vi "Pressures_Low_Server.vi"(0 "Serial port":refnum<visa-resource-name>="COM1", 1 "Commands":T2[](array[typedef]), 5 "Data rate (Hz)":dbl=100.0, 7 "Max. num. sensors (override)":u8=64 max=64, 9 "Wait for HW trigger":bool, 11 "Finite samples":bool=TRUE, 12 "N samples":u32=1000, 14 "Error in":errorcluster) -> (4 "P data (mode 0)":T8[](array[typedef]), 15 "Error out":errorcluster)   [LabVIEW 2020]
doc: "User interface for 64 pressure multiplexer system designed by Paul Nathan, 02/2016"
uses:
  Ctls/System status.ctl
  Ctls/Environmental state values.ctl
  Ctls/Inertial state values.ctl
  Ctls/AccelGyro constants.ctl
  Ctls/Pressure sensor constants.ctl
  Ctls/Cmd list.ctl
  Ctls/Data values, Mode 0 (for datalog).ctl
  Ctls/All state values (for datalog).ctl
  Ctls/Cmd str.ctl
  Ctls/Data values, Mode 1 (for datalog).ctl
  Pressure_Multiplexer_Server_Global.vi
panel:
  in  "Main tabs":T1(tab)
  in  "Env. period (ms)":i32=1000 min=0
  out "Command":T2
  out "ACK 8":bool caption="ACK"
  out "ACK 7":bool caption="ACK"
  out "ACK 6":bool caption="ACK"
  out "AccelGyro constants":T3={"gyrRange"=125.0, "accRange"=2.0, "gx offset"=0.0, "gy offset"=0.0, "gz offset"=0.0, "ax offset"=0.0, "ay offset"=0.0, "az offset"=0.0, "axyz scale"=1.0} {"axyz scale" format="%#_4f"; "az offset" format="%#_4f"; "ay offset" format="%#_4f"; "ax offset" format="%#_4f"; "gz offset" format="%#_4f"; "gy offset" format="%#_4f"; "gx offset" format="%#_4f"; "gyrRange" format="%#_4f"; "accRange" format="%#_4f"}
  out "Faulty sensors":i32[](array[numeric])
  out "ACK 5":bool caption="ACK"
  out "Active sensors":i32[](array[numeric])
  out "ACK 4":bool caption="ACK"
  in  "Gyro. rate (Hz)":u8(ring) items=["6.25", "12.5", "25", "50", "100", "200", "400", "800", "1600", "3200"]
  in  "Gyro. range (dps)":u8(ring) items=["+/- 125", "+/- 250", "+/- 500", "+/- 1000", "+/- 2000"]
  in  "Accel. rate (Hz)":u8(ring)=1 items=["3.125", "6.25", "12.5", "25", "50", "100", "200", "400", "800", "1600"]
  in  "Accel. range (g)":u8(ring) items=["+/- 2", "+/- 4", "+/- 8", "+/- 16"]
  out "Inertial state values":T4 {"w_z (dps)" format="%#_4f"; "a_y (g)" format="%#_4f"; "a_z (g)" format="%#_4f"; "w_y (dps)" format="%#_4f"; "a_x (g)" format="%#_4f"; "Sensor temp. (degC)" format="%#.2f"; "w_x (dps)" format="%#_4f"}
  out "Environmental state values":T5 {"Dew point (degC)" format="%#.2f"; "Density (kg/m^3)" format="%#.3f"; "Pressure alt. (m)" format="%#.2f"; "Density alt. (m)" format="%#.2f"; "Rel. Humidity (%)" format="%#.2f"; "P_atmos (Pa)" format="%#_6f"; "Sensor temp. (degC)" format="%#.2f"; "Thermistor (degC)" format="%#.2f"}
  out "System status":T6
  out "ACK 3":bool caption="ACK"
  out "ACK 1":bool caption="ACK"
  in  "Data mode":u8(ring) items=["P", "P & T"]
  out "ACK 2":bool caption="ACK"
  out "Main Power":bool
  out "L_data (bytes)":u16
  out "Serial no.":u16 format="%04x"
  out "Active pressure sensor constants":T7[](array[typedef])
  out "No Of Channels":i32=1000
  out "Streaming":bool
  out "Clock drift":bool
  out "Sensor temperatures time trace (Mode \"P & T\" only)":sgl[][](graph)
  out "Pressures time trace":sgl[][](graph)
  in  "Stop streaming":bool
  out "Stale samples flag":u8[][](graph)
  out "Samples acquired":u32
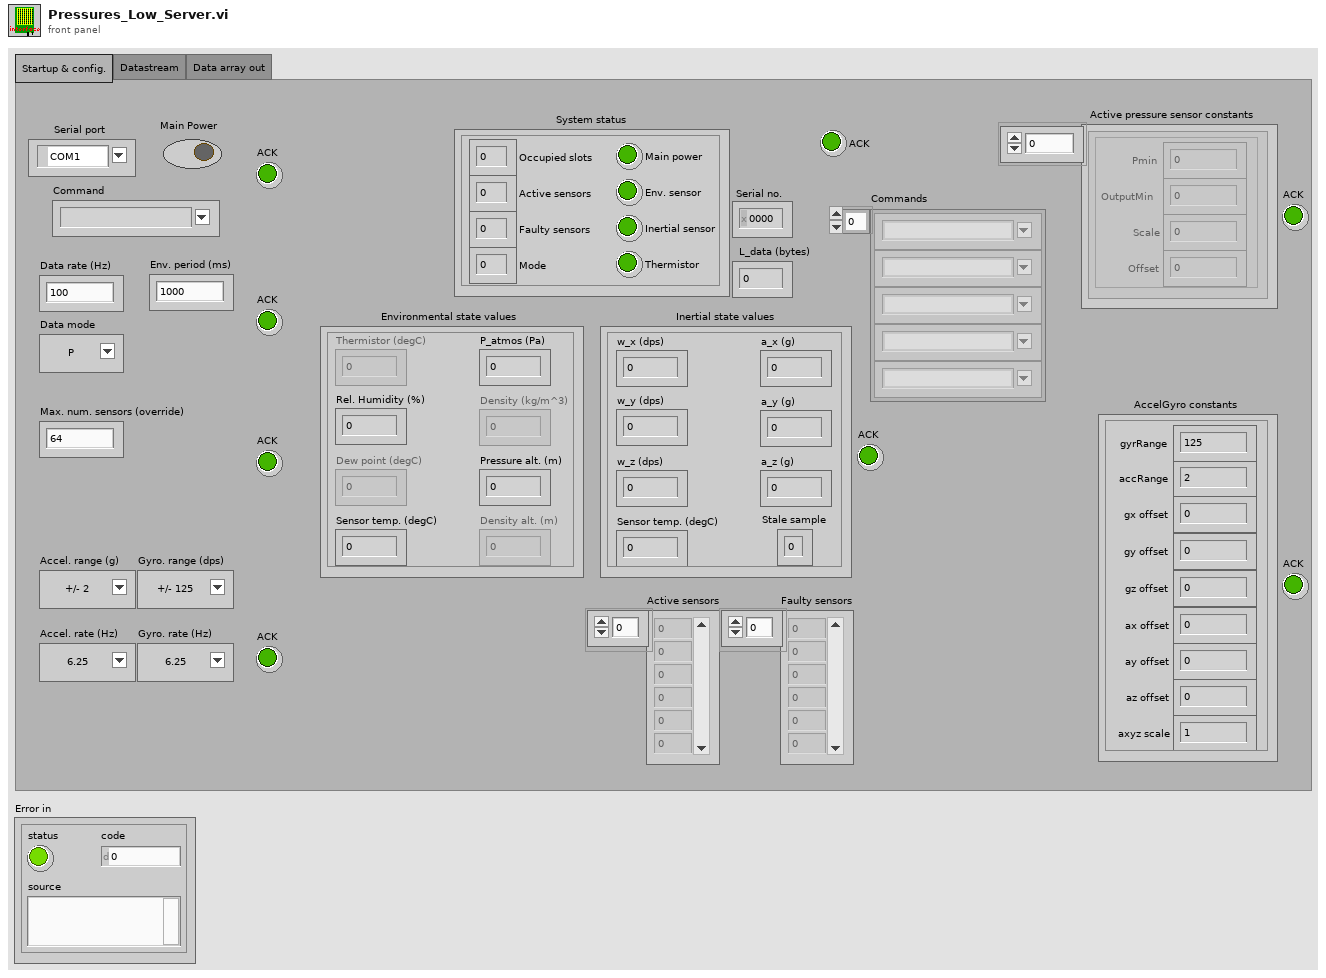
[diagram p1: front panel]
types:
  T1 = enum32{"Startup & config.", "Datastream", "Data array out"}
  T2 = typedef "Cmd list.ctl" = string
  T3 = typedef "AccelGyro constants.ctl" = cluster{"gyrRange":sgl, "accRange":sgl, "gx offset":sgl, "gy offset":sgl, "gz offset":sgl, "ax offset":sgl, "ay offset":sgl, "az offset":sgl, "axyz scale":sgl}
  T4 = typedef "Inertial state values.ctl" = cluster{"w_x (dps)":sgl, "w_y (dps)":sgl, "w_z (dps)":sgl, "a_x (g)":sgl, "a_y (g)":sgl, "a_z (g)":sgl, "Stale sample":u8, "Sensor temp. (degC)":sgl}
  T5 = typedef "Environmental state values.ctl" = cluster{"Thermistor (degC)":sgl, "Sensor temp. (degC)":sgl, "P_atmos (Pa)":sgl, "Rel. Humidity (%)":sgl, "Density (kg/m^3)":sgl, "Dew point (degC)":sgl, "Pressure alt. (m)":sgl, "Density alt. (m)":sgl}
  T6 = typedef "System status.ctl" = cluster{"Main power":bool, "Occupied slots":u8, "Active sensors":u8, "Faulty sensors":u8, "Env. sensor":bool, "Inertial sensor":bool, "Thermistor":bool, "Mode":u8}
  T7 = typedef "Pressure sensor constants.ctl" = cluster{"Pmin":sgl, "OutputMin":sgl, "Scale":sgl, "Offset":sgl}
  T8 = typedef "Data values, Mode 0 (for datalog).ctl" = cluster{"Time Stamp":timestamp, "dt (us)":sgl, "dt_warn":u8, "Pressures":sgl[], "Statuses":u8[]}
  T9 = typedef "All state values (for datalog).ctl" = cluster{"Time Stamp":timestamp, "dt (ms)":i32, "Environmental state values":T5, "Inertial state values":T4}
  T10 = typedef "Cmd str.ctl" = string
  T11 = typedef "Data values, Mode 1 (for datalog).ctl" = cluster{"Time Stamp":timestamp, "dt (us)":sgl, "dt_warn":u8, "Pressures":sgl[], "Die temps.":sgl[], "Statuses":u8[]}
  T12 = enum8{"Enabled", "Disabled", "Disabled and Grayed Out"}
  T13 = typedef "Rendezvous RefNum" = refnum<k1>
  T14 = typedef "EEPROM page.ctl" = cluster{"Pmin (Pa)":sgl, "Pmax (Pa)":sgl, "maxCount":u16, "minCount":u16, "Poffset (Pa)":sgl}
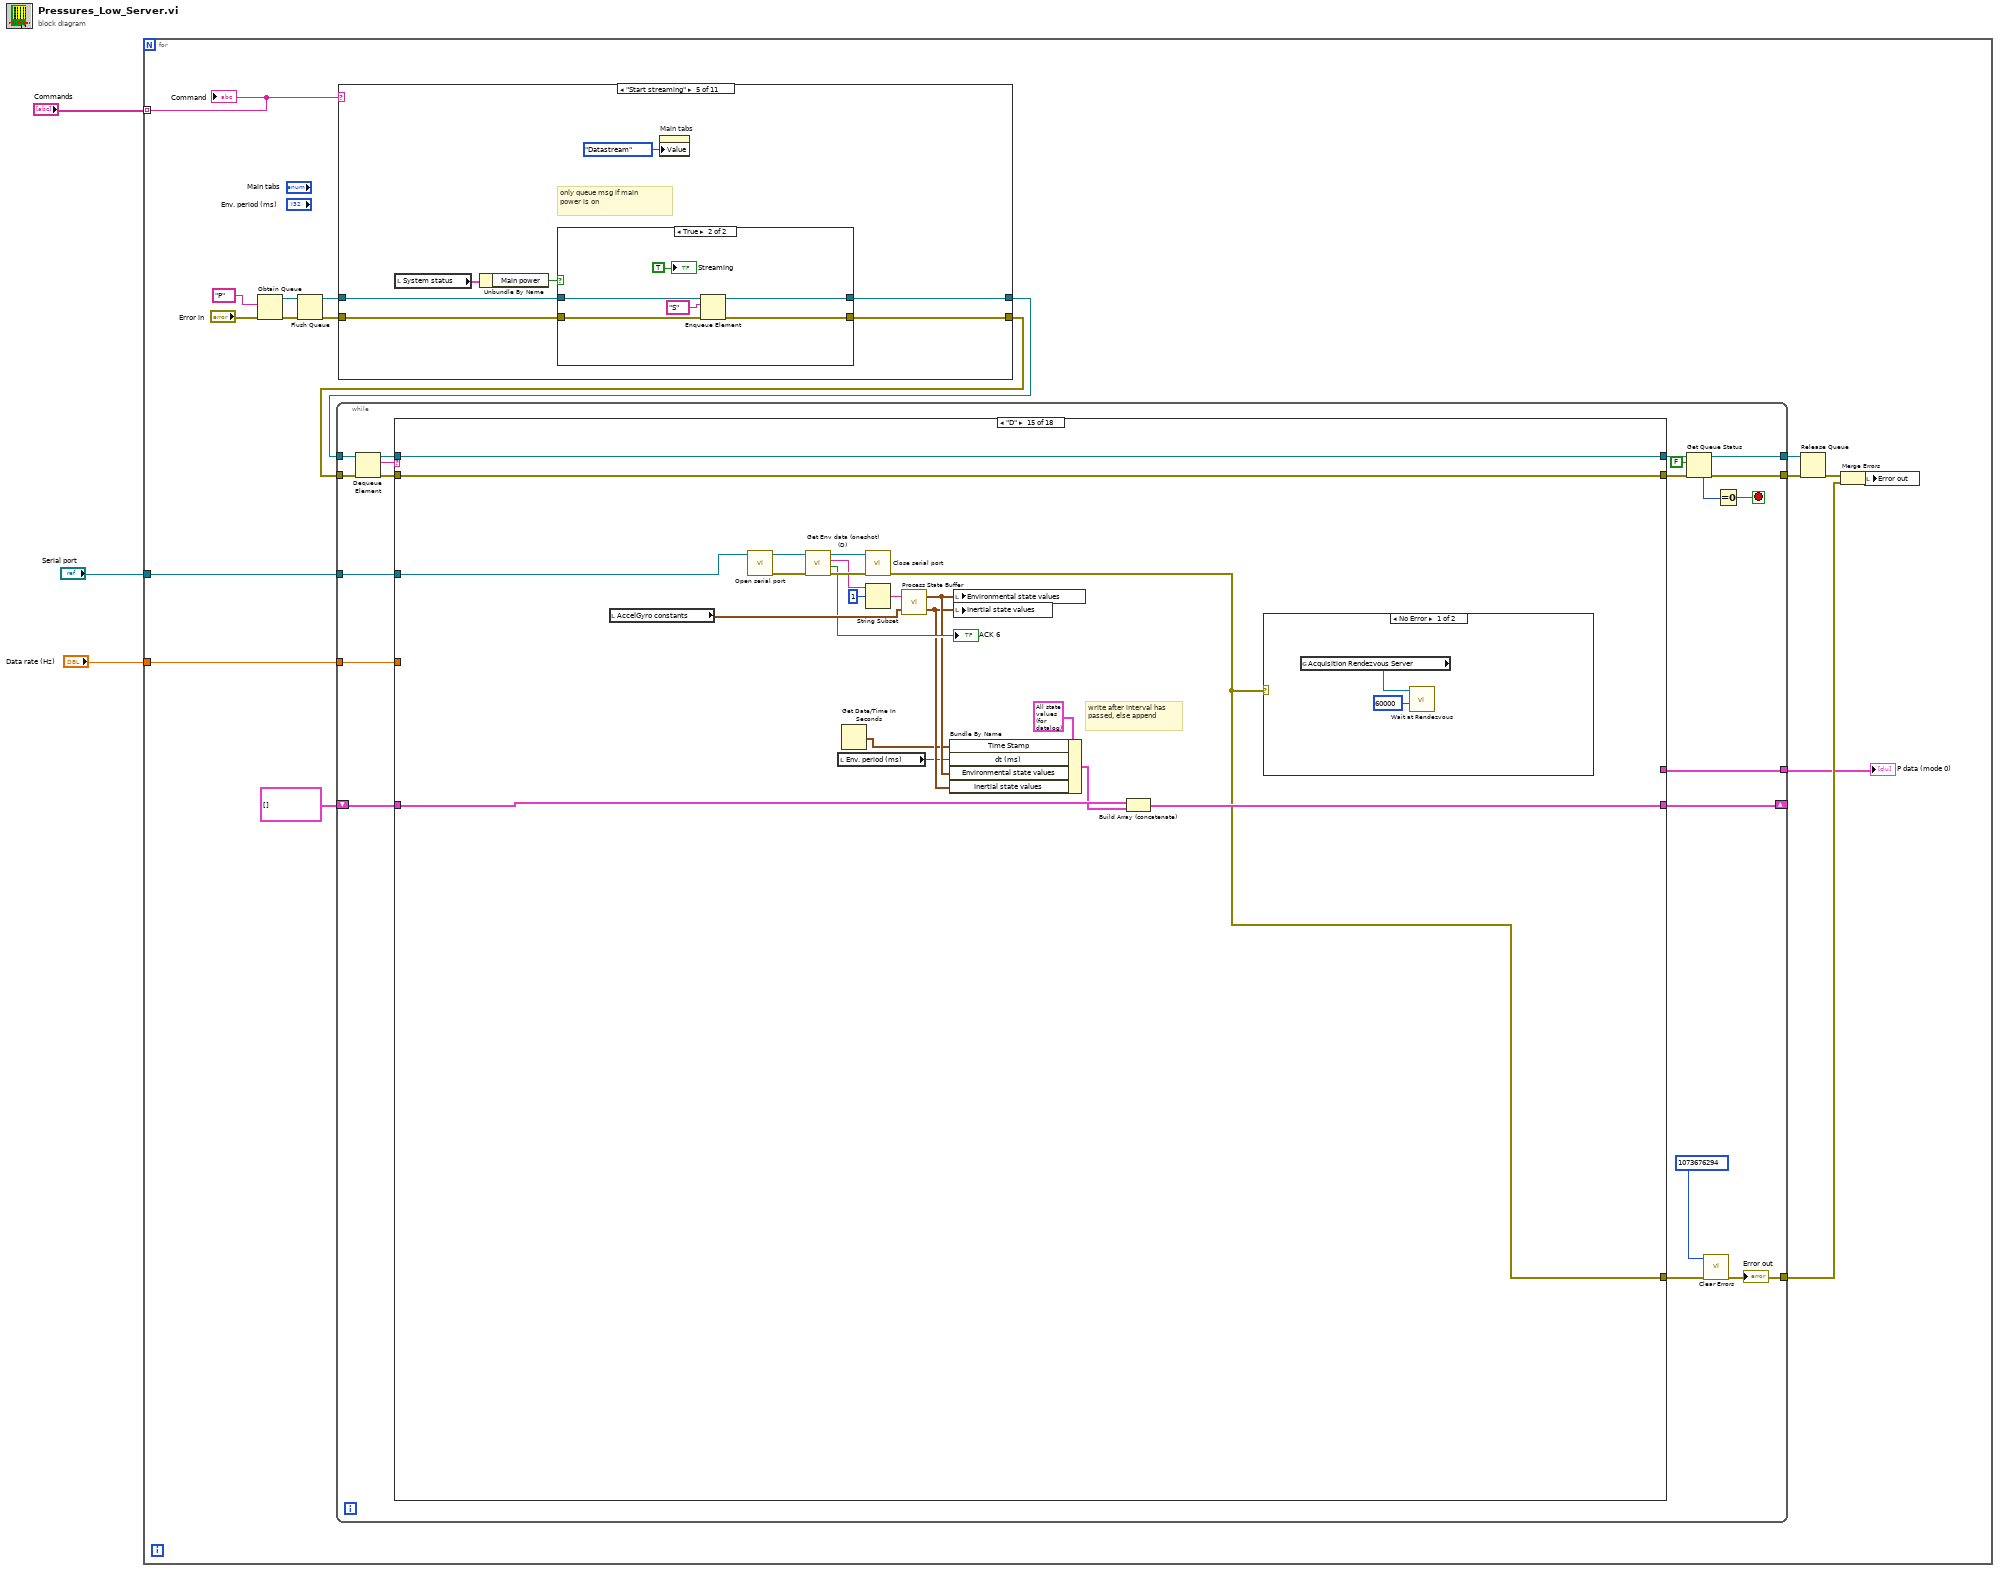
[diagram p0: block diagram]
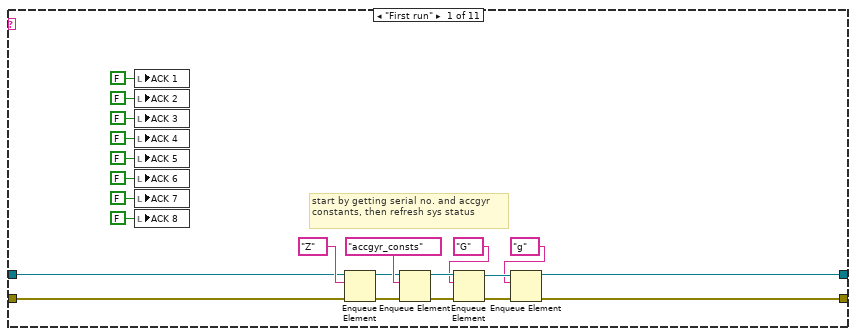
[diagram p2: hidden frame]
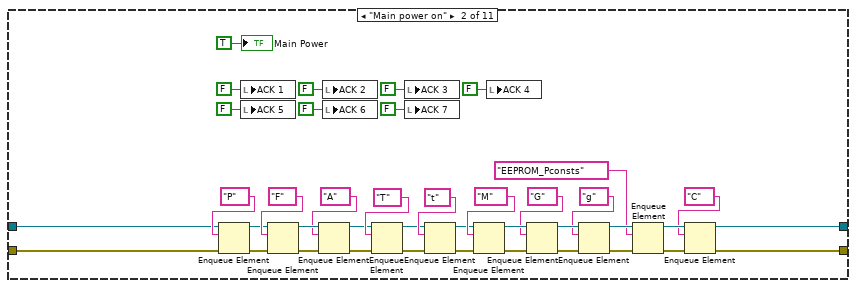
[diagram p3: hidden frame]
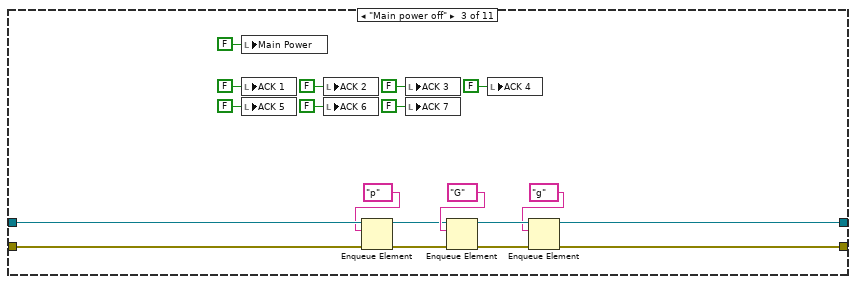
[diagram p4: hidden frame]
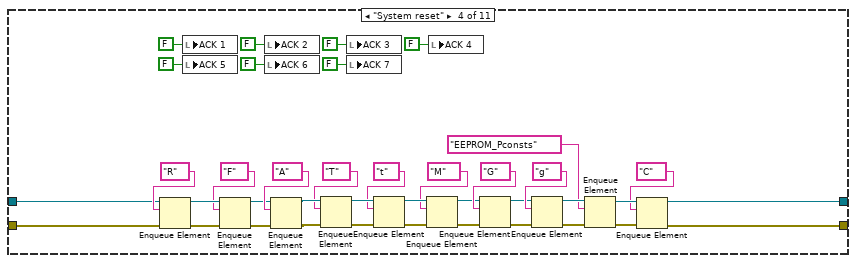
[diagram p5: hidden frame]
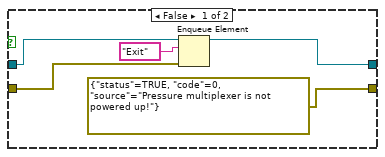
[diagram p6: hidden frame]
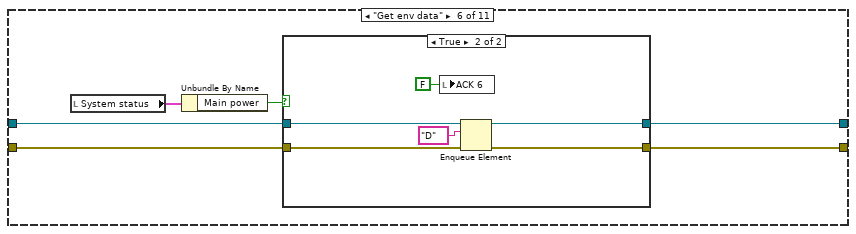
[diagram p7: hidden frame]
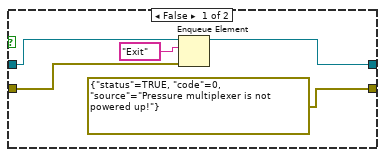
[diagram p8: hidden frame]
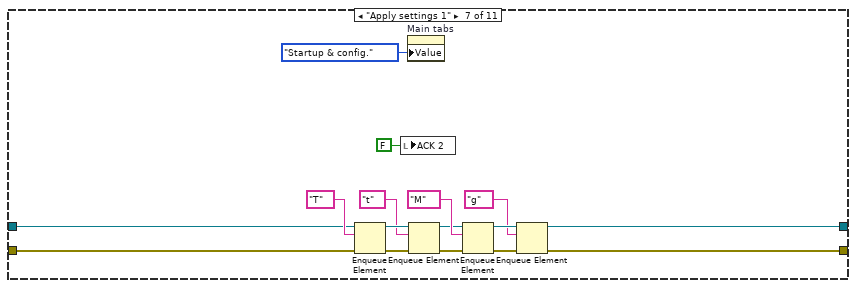
[diagram p9: hidden frame]
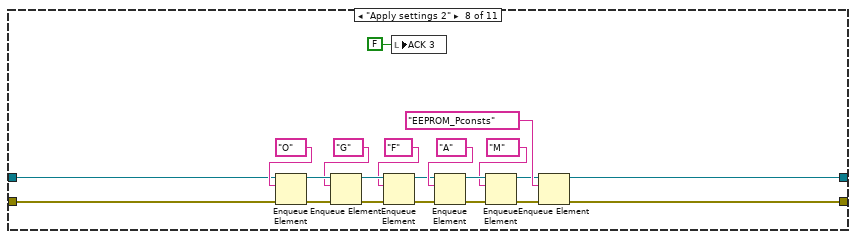
[diagram p10: hidden frame]
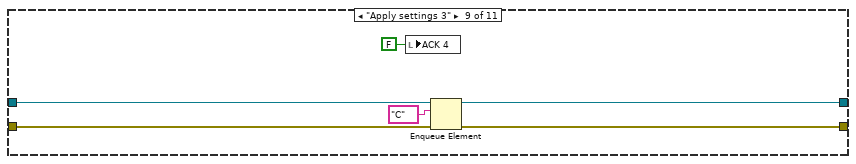
[diagram p11: hidden frame]
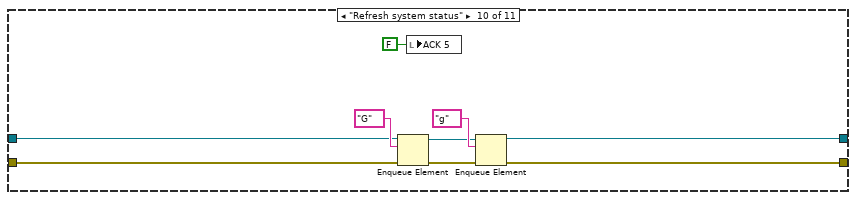
[diagram p12: hidden frame]
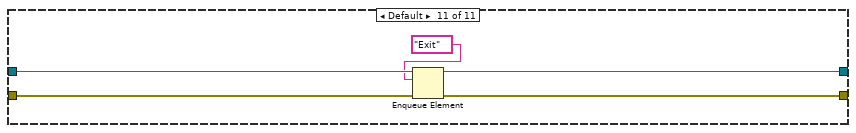
[diagram p13: hidden frame]
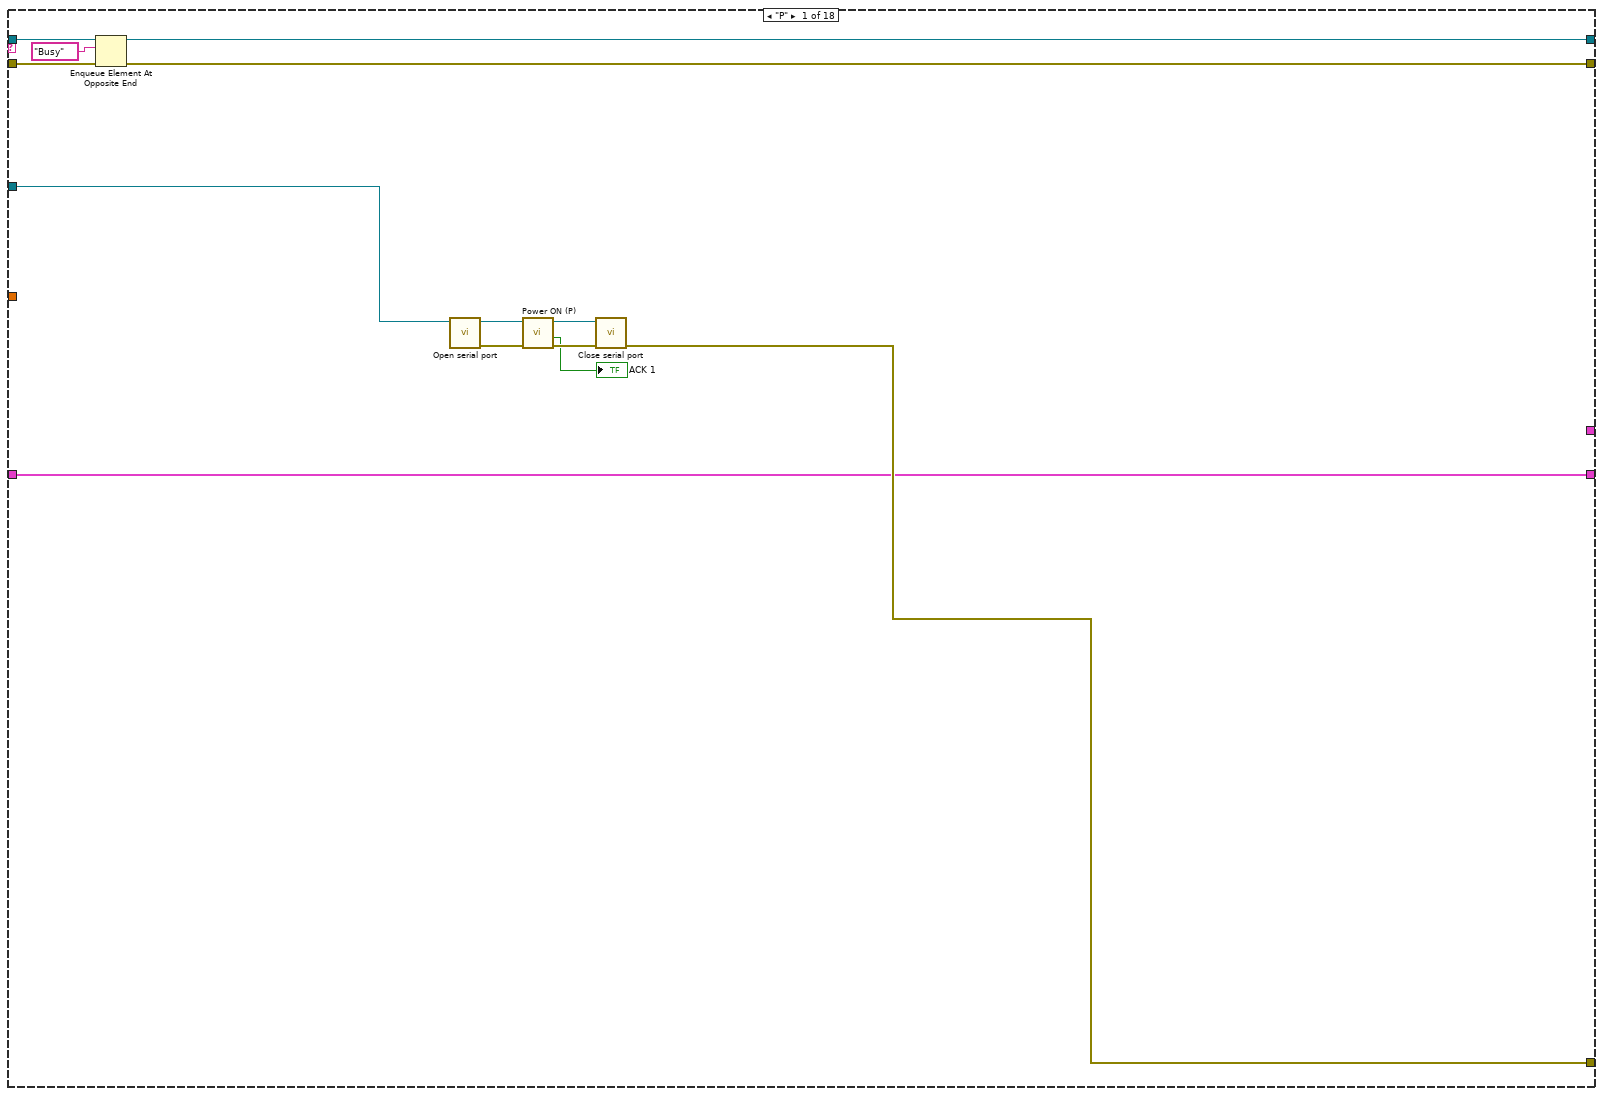
[diagram p14: hidden frame]
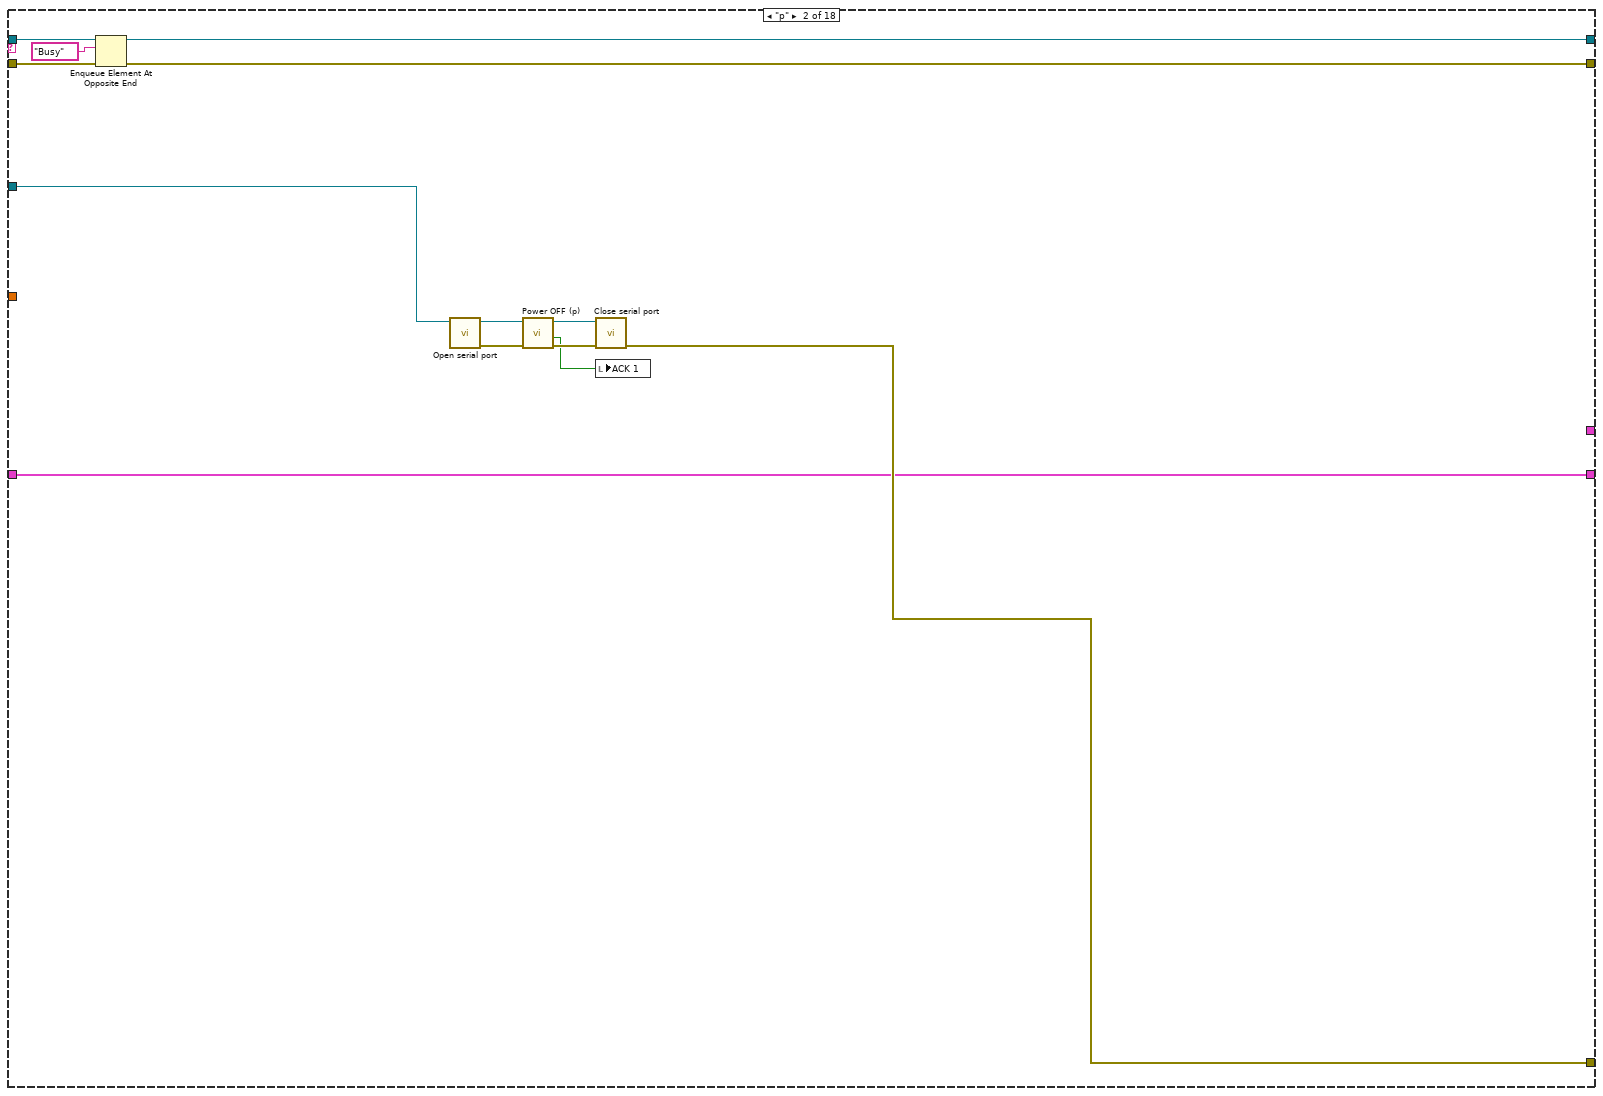
[diagram p15: hidden frame]
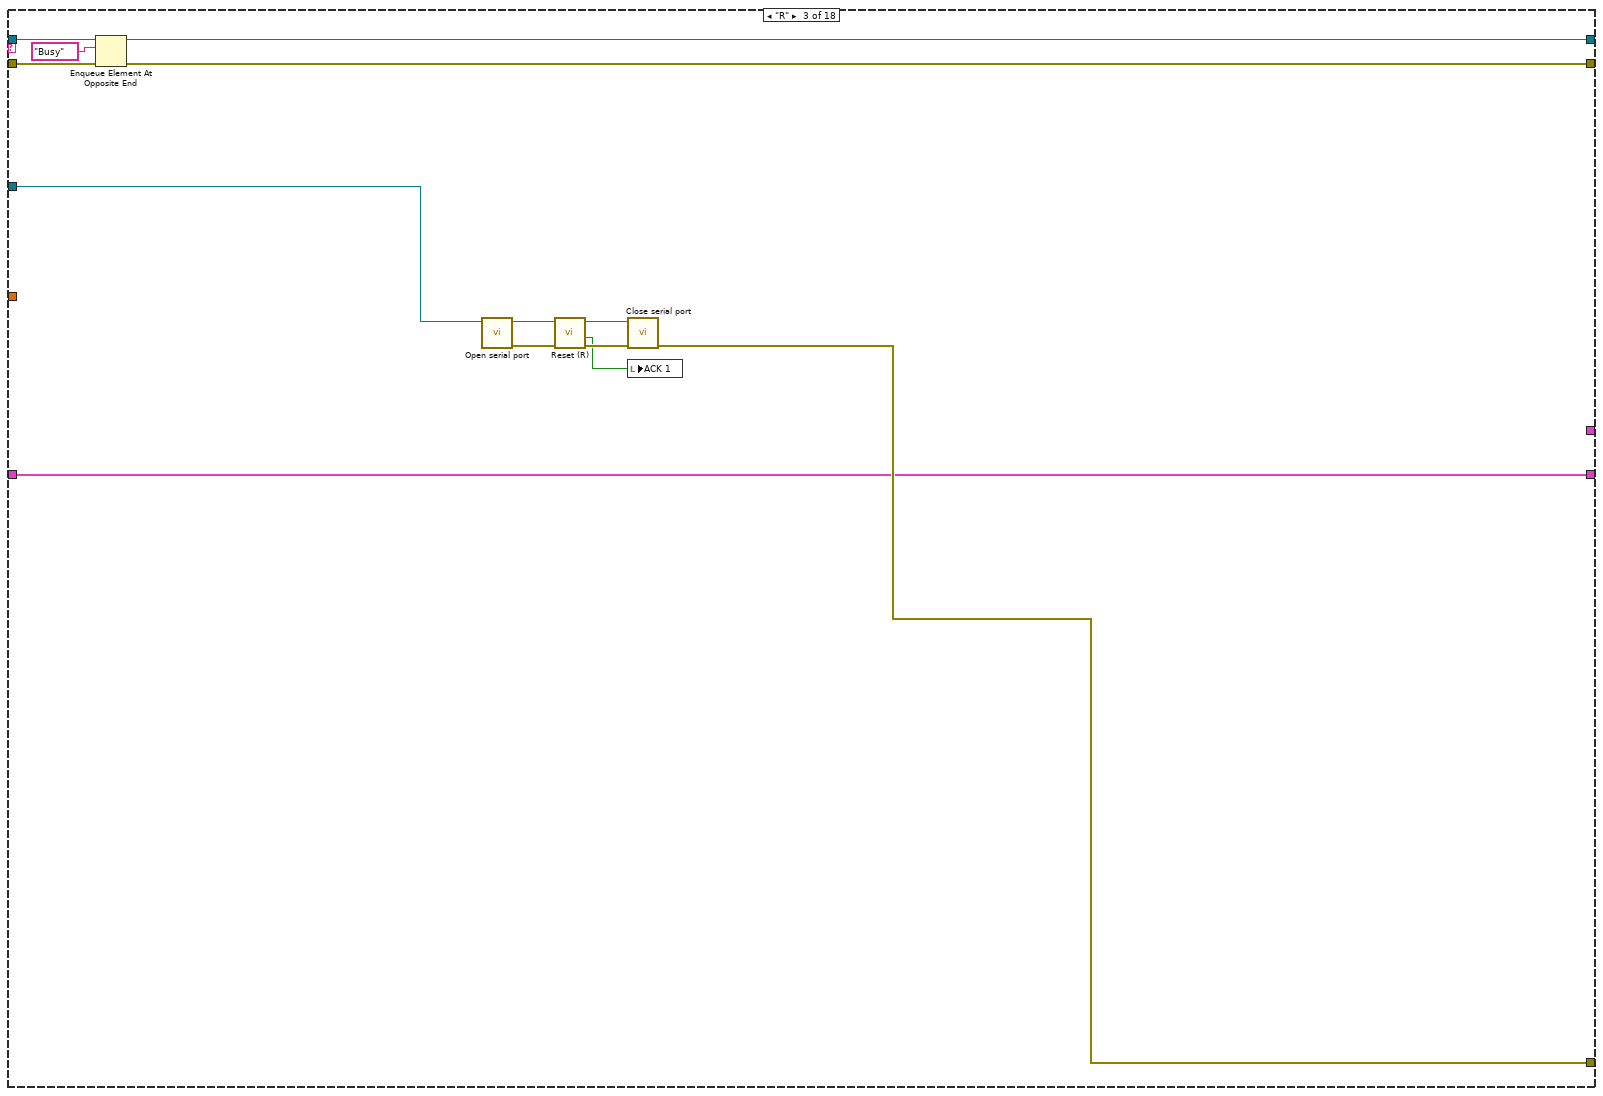
[diagram p16: hidden frame]
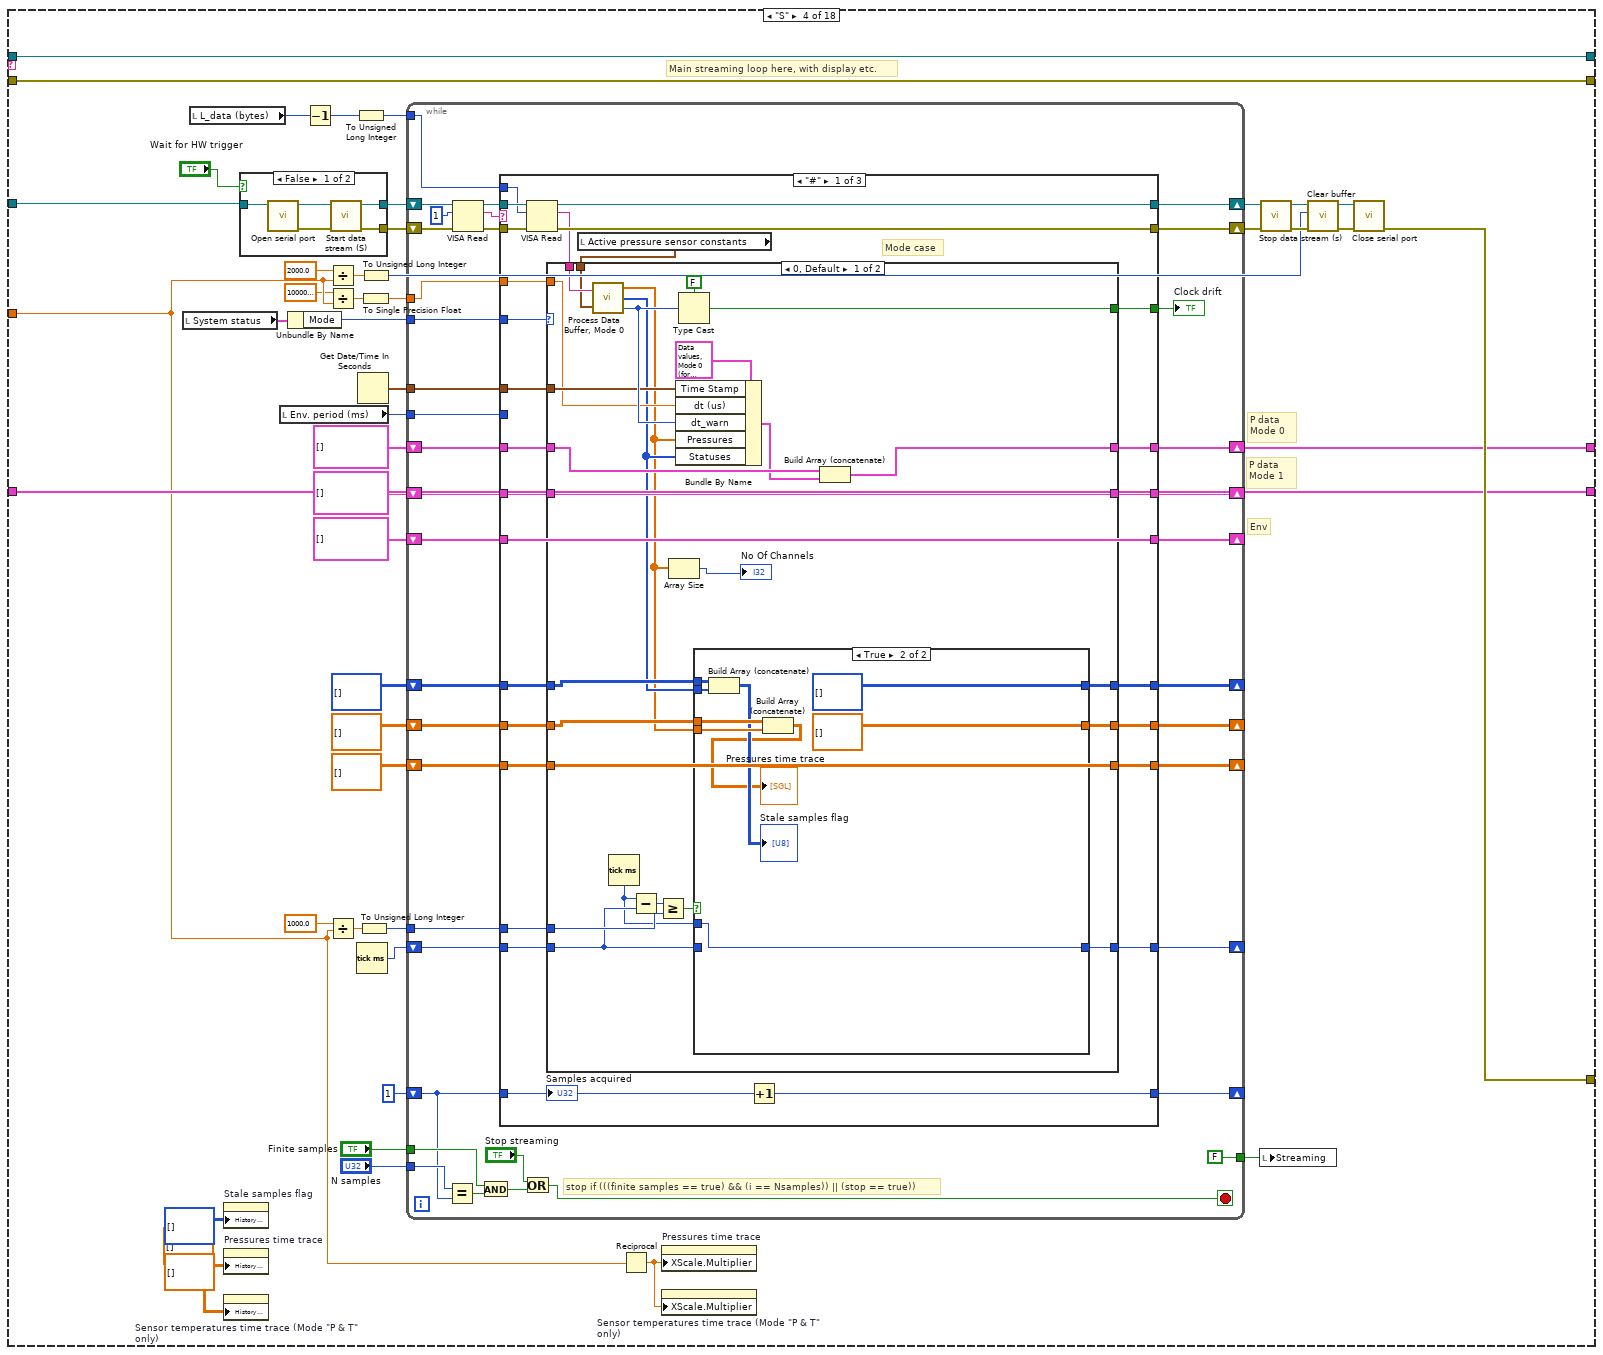
[diagram p17: hidden frame]
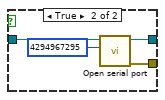
[diagram p18: hidden frame]
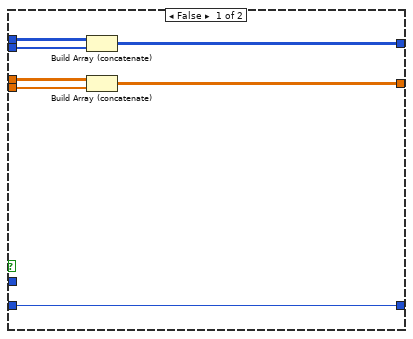
[diagram p19: hidden frame]
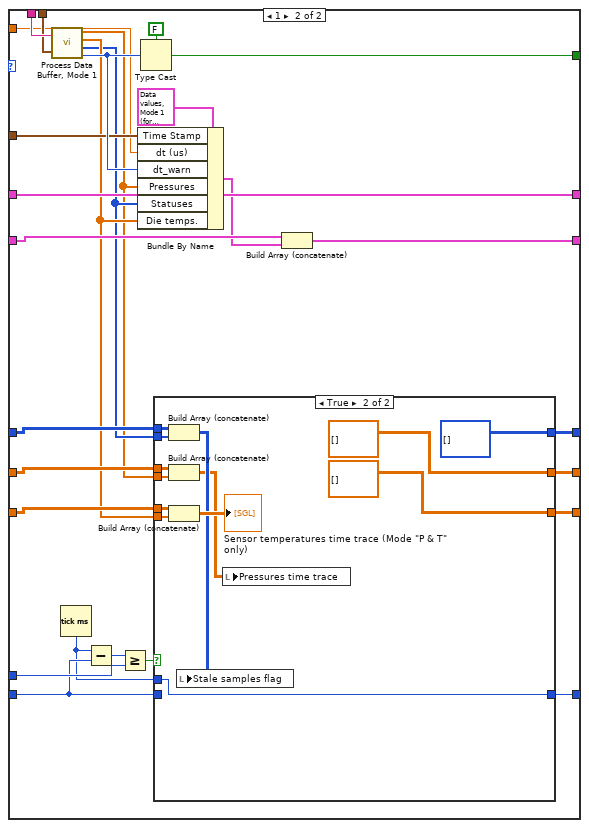
[diagram p20: hidden frame]
diagram:
  n1 = for {
    tunnel: "Serial port" -> [w6]
    tunnel: "Data rate (Hz)" -> [w5]
    tunnel: "Commands" -> [w4] mode=indexing
    n2 = Obtain Queue(element data type=T10 "P" ("Cmd"), error in (no error)="Error in") -> (queue out=w21:refnum<queue>, error out=w20:errorcluster)  [unwired: 3 in, 1 out]
    n3 = Flush Queue(queue=w21, error in (no error)=w20) -> (queue out=w10:refnum<queue>, error out=w9:errorcluster)  [unwired: 1 out]
    n4 = case shown="\"Start streaming\"" w4 {
      tunnel: [w31 w54 w94 w111 w143 w162 w180 w195 w216 w221 w229] -> w12
      tunnel: w9 -> [w32 w81 w101 w112 w146 w163 w181 w196 w217 w224 w233]
      tunnel: w10 -> [w33 w82 w102 w113 w145 w164 w182 w197 w218 w223 w232]
      tunnel: [w30 w53 w93 w110 w144 w161 w179 w194 w215 w222 w230] -> w11
      frame "First run" {
        # "start by getting serial no. and accgyr constants, then refresh sys status"
        n5 = local write "ACK 1"(FALSE ("ACK 8")) -> ()
        n6 = local write "ACK 2"(FALSE ("ACK 6")) -> ()
        n7 = local write "ACK 3"(FALSE ("ACK 8")) -> ()
        n8 = local write "ACK 4"(FALSE ("Done")) -> ()
        n9 = local write "ACK 5"(FALSE ("ACK 8")) -> ()
        n10 = local write "ACK 6"(FALSE ("ACK 6")) -> ()
        n11 = local write "ACK 7"(FALSE ("ACK 6")) -> ()
        n12 = local write "ACK 8"(FALSE ("ACK 8")) -> ()
        n13 = Enqueue Element(queue=w33, element=T10 "Z", error in (no error)=w32) -> (queue out=w35:refnum<queue>, error out=w36:errorcluster)  [unwired: 1 in, 1 out]
        n14 = Enqueue Element(queue=w35, element=T10 "accgyr_consts", error in (no error)=w36) -> (queue out=w42:refnum<queue>, error out=w43:errorcluster)  [unwired: 1 in, 1 out]
        n15 = Enqueue Element(queue=w42, element=T10 "G" ("Cmd"), error in (no error)=w43) -> (queue out=w40:refnum<queue>, error out=w39:errorcluster)  [unwired: 1 in, 1 out]
        n16 = Enqueue Element(queue=w40, element=T10 "g" ("Cmd"), error in (no error)=w39) -> (queue out=w30:refnum<queue>, error out=w31:errorcluster)  [unwired: 1 in, 1 out]
      }
      frame "Main power on" {
        n17 = Enqueue Element(queue=w82, element=T10 "P" ("Cmd"), error in (no error)=w81) -> (queue out=w75:refnum<queue>, error out=w74:errorcluster)  [unwired: 1 in, 1 out]
        n18 = local write "ACK 1"(FALSE ("ACK 1")) -> ()
        n19 = local write "ACK 5"(FALSE ("ACK 8")) -> ()
        n20 = Enqueue Element(queue=w75, element=T10 "F" ("Cmd"), error in (no error)=w74) -> (queue out=w79:refnum<queue>, error out=w80:errorcluster)  [unwired: 1 in, 1 out]
        n21 = Enqueue Element(queue=w79, element=T10 "A" ("Cmd"), error in (no error)=w80) -> (queue out=w60:refnum<queue>, error out=w59:errorcluster)  [unwired: 1 in, 1 out]
        n22 = local write "ACK 2"(FALSE ("ACK 6")) -> ()
        n23 = local write "ACK 6"(FALSE ("ACK 6")) -> ()
        n24 = Enqueue Element(queue=w60, element=T10 "T" ("Cmd"), error in (no error)=w59) -> (queue out=w62:refnum<queue>, error out=w61:errorcluster)  [unwired: 1 in, 1 out]
        n25 = local write "ACK 3"(FALSE ("ACK 8")) -> ()
        n26 = local write "ACK 7"(FALSE ("ACK 6")) -> ()
        n27 = Enqueue Element(queue=w62, element=T10 "t" ("Cmd"), error in (no error)=w61) -> (queue out=w57:refnum<queue>, error out=w58:errorcluster)  [unwired: 1 in, 1 out]
        n28 = Enqueue Element(queue=w57, element=T10 "M" ("Cmd"), error in (no error)=w58) -> (queue out=w71:refnum<queue>, error out=w70:errorcluster)  [unwired: 1 in, 1 out]
        n29 = local write "ACK 4"(FALSE ("Done")) -> ()
        n30 = Enqueue Element(queue=w71, element=T10 "G" ("Cmd"), error in (no error)=w70) -> (queue out=w72:refnum<queue>, error out=w73:errorcluster)  [unwired: 1 in, 1 out]
        n31 = Enqueue Element(queue=w72, element=T10 "g" ("Cmd"), error in (no error)=w73) -> (queue out=w67:refnum<queue>, error out=w66:errorcluster)  [unwired: 1 in, 1 out]
        n32 = Enqueue Element(queue=w67, element=T10 "EEPROM_Pconsts" ("Cmd"), error in (no error)=w66) -> (queue out=w56:refnum<queue>, error out=w55:errorcluster)  [unwired: 1 in, 1 out]
        n33 = Enqueue Element(queue=w56, element=T10 "C" ("Cmd"), error in (no error)=w55) -> (queue out=w53:refnum<queue>, error out=w54:errorcluster)  [unwired: 1 in, 1 out]
        "Main Power" <- TRUE ("Main Power")
      }
      frame "Main power off" {
        n34 = local write "Main Power"(FALSE ("Main Power")) -> ()
        n35 = local write "ACK 1"(FALSE ("ACK 1")) -> ()
        n36 = local write "ACK 5"(FALSE ("ACK 8")) -> ()
        n37 = local write "ACK 2"(FALSE ("ACK 6")) -> ()
        n38 = local write "ACK 6"(FALSE ("ACK 6")) -> ()
        n39 = Enqueue Element(queue=w102, element=T10 "p" ("Cmd"), error in (no error)=w101) -> (queue out=w98:refnum<queue>, error out=w97:errorcluster)  [unwired: 1 in, 1 out]
        n40 = local write "ACK 3"(FALSE ("ACK 8")) -> ()
        n41 = local write "ACK 7"(FALSE ("ACK 6")) -> ()
        n42 = Enqueue Element(queue=w98, element=T10 "G" ("Cmd"), error in (no error)=w97) -> (queue out=w96:refnum<queue>, error out=w95:errorcluster)  [unwired: 1 in, 1 out]
        n43 = local write "ACK 4"(FALSE ("Done")) -> ()
        n44 = Enqueue Element(queue=w96, element=T10 "g" ("Cmd"), error in (no error)=w95) -> (queue out=w93:refnum<queue>, error out=w94:errorcluster)  [unwired: 1 in, 1 out]
      }
      frame "System reset" {
        n45 = Enqueue Element(queue=w113, element=T10 "R" ("Cmd"), error in (no error)=w112) -> (queue out=w125:refnum<queue>, error out=w126:errorcluster)  [unwired: 1 in, 1 out]
        n46 = local write "ACK 1"(FALSE ("ACK 1")) -> ()
        n47 = local write "ACK 5"(FALSE ("ACK 8")) -> ()
        n48 = Enqueue Element(queue=w125, element=T10 "F" ("Cmd"), error in (no error)=w126) -> (queue out=w117:refnum<queue>, error out=w127:errorcluster)  [unwired: 1 in, 1 out]
        n49 = local write "ACK 2"(FALSE ("ACK 6")) -> ()
        n50 = local write "ACK 6"(FALSE ("ACK 6")) -> ()
        n51 = Enqueue Element(queue=w117, element=T10 "A" ("Cmd"), error in (no error)=w127) -> (queue out=w135:refnum<queue>, error out=w136:errorcluster)  [unwired: 1 in, 1 out]
        n52 = Enqueue Element(queue=w135, element=T10 "T" ("Cmd"), error in (no error)=w136) -> (queue out=w133:refnum<queue>, error out=w134:errorcluster)  [unwired: 1 in, 1 out]
        n53 = local write "ACK 3"(FALSE ("ACK 8")) -> ()
        n54 = local write "ACK 7"(FALSE ("ACK 6")) -> ()
        n55 = Enqueue Element(queue=w133, element=T10 "t" ("Cmd"), error in (no error)=w134) -> (queue out=w137:refnum<queue>, error out=w138:errorcluster)  [unwired: 1 in, 1 out]
        n56 = Enqueue Element(queue=w137, element=T10 "M" ("Cmd"), error in (no error)=w138) -> (queue out=w121:refnum<queue>, error out=w128:errorcluster)  [unwired: 1 in, 1 out]
        n57 = local write "ACK 4"(FALSE ("Done")) -> ()
        n58 = Enqueue Element(queue=w121, element=T10 "G" ("Cmd"), error in (no error)=w128) -> (queue out=w120:refnum<queue>, error out=w129:errorcluster)  [unwired: 1 in, 1 out]
        n59 = Enqueue Element(queue=w120, element=T10 "g" ("Cmd"), error in (no error)=w129) -> (queue out=w124:refnum<queue>, error out=w130:errorcluster)  [unwired: 1 in, 1 out]
        n60 = Enqueue Element(queue=w124, element=T10 "EEPROM_Pconsts" ("Cmd"), error in (no error)=w130) -> (queue out=w140:refnum<queue>, error out=w141:errorcluster)  [unwired: 1 in, 1 out]
        n61 = Enqueue Element(queue=w140, element=T10 "C" ("Cmd"), error in (no error)=w141) -> (queue out=w110:refnum<queue>, error out=w111:errorcluster)  [unwired: 1 in, 1 out]
      }
      frame "Start streaming" {
        # "only queue msg if main power is on"
        n62 = local read "System status"() -> (w148:T6)
        n63 = Unbundle By Name(w148) -> ("Main power"=w147:bool)
        n64 = case shown="True" w147 {
          tunnel: w145 -> [w151 w158]
          tunnel: w146 -> [w149 w157]
          tunnel: [w150 w155] -> w144
          tunnel: [errorcluster {"status"=TRUE, "code"=0, "source"="Pressure multiplexer is not powered up!"} ("error out") w156] -> w143
          frame False {
            n65 = Enqueue Element(queue=w151, element=T10 "Exit" ("Cmd"), error in (no error)=w149) -> (queue out=w150:refnum<queue>)  [unwired: 1 in, 2 out]
          }
          frame True {
            n66 = Enqueue Element(queue=w158, element=T10 "S" ("Cmd"), error in (no error)=w157) -> (queue out=w155:refnum<queue>, error out=w156:errorcluster)  [unwired: 1 in, 1 out]
            "Streaming" <- TRUE ("Streaming")
          }
        }
        n67 = property on="Main tabs" class="TabCtl (strict)"("Value"=T1."Datastream" ("Main tabs")) -> ()  [unwired: 2 in, 2 out]
      }
      frame "Get env data" {
        n68 = local read "System status"() -> (w165:T6)
        n69 = Unbundle By Name(w165) -> ("Main power"=w160:bool)
        n70 = case shown="True" w160 {
          tunnel: w164 -> [w168 w175]
          tunnel: w163 -> [w166 w174]
          tunnel: [w167 w172] -> w161
          tunnel: [errorcluster {"status"=TRUE, "code"=0, "source"="Pressure multiplexer is not powered up!"} ("error out") w173] -> w162
          frame False {
            n71 = Enqueue Element(queue=w168, element=T10 "Exit" ("Cmd"), error in (no error)=w166) -> (queue out=w167:refnum<queue>)  [unwired: 1 in, 2 out]
          }
          frame True {
            n72 = local write "ACK 6"(FALSE ("ACK 6")) -> ()
            n73 = Enqueue Element(queue=w175, element=T10 "D" ("Cmd"), error in (no error)=w174) -> (queue out=w172:refnum<queue>, error out=w173:errorcluster)  [unwired: 1 in, 1 out]
          }
        }
      }
      frame "Apply settings 1" {
        n74 = Enqueue Element(queue=w182, element=T10 "T" ("Cmd"), error in (no error)=w181) -> (queue out=w185:refnum<queue>, error out=w186:errorcluster)  [unwired: 1 in, 1 out]
        n75 = local write "ACK 2"(FALSE ("ACK 6")) -> ()
        n76 = property on="Main tabs" class="TabCtl (strict)"("Value"=T1."Startup & config." ("Main tabs")) -> ()  [unwired: 2 in, 2 out]
        n77 = Enqueue Element(queue=w185, element=T10 "t" ("Cmd"), error in (no error)=w186) -> (queue out=w188:refnum<queue>, error out=w187:errorcluster)  [unwired: 1 in, 1 out]
        n78 = Enqueue Element(queue=w188, element=T10 "M" ("Cmd"), error in (no error)=w187) -> (queue out=w191:refnum<queue>, error out=w192:errorcluster)  [unwired: 1 in, 1 out]
        n79 = Enqueue Element(queue=w191, element=T10 "g" ("Cmd"), error in (no error)=w192) -> (queue out=w179:refnum<queue>, error out=w180:errorcluster)  [unwired: 1 in, 1 out]
      }
      frame "Apply settings 2" {
        n80 = Enqueue Element(queue=w197, element=T10 "O" ("Cmd"), error in (no error)=w196) -> (queue out=w200:refnum<queue>, error out=w201:errorcluster)  [unwired: 1 in, 1 out]
        n81 = Enqueue Element(queue=w200, element=T10 "G" ("Cmd"), error in (no error)=w201) -> (queue out=w212:refnum<queue>, error out=w213:errorcluster)  [unwired: 1 in, 1 out]
        n82 = Enqueue Element(queue=w212, element=T10 "F" ("Cmd"), error in (no error)=w213) -> (queue out=w208:refnum<queue>, error out=w207:errorcluster)  [unwired: 1 in, 1 out]
        n83 = local write "ACK 3"(FALSE ("ACK 8")) -> ()
        n84 = Enqueue Element(queue=w208, element=T10 "A" ("Cmd"), error in (no error)=w207) -> (queue out=w210:refnum<queue>, error out=w211:errorcluster)  [unwired: 1 in, 1 out]
        n85 = Enqueue Element(queue=w210, element=T10 "M" ("Cmd"), error in (no error)=w211) -> (queue out=w203:refnum<queue>, error out=w202:errorcluster)  [unwired: 1 in, 1 out]
        n86 = Enqueue Element(queue=w203, element=T10 "EEPROM_Pconsts" ("Cmd"), error in (no error)=w202) -> (queue out=w194:refnum<queue>, error out=w195:errorcluster)  [unwired: 1 in, 1 out]
      }
      frame "Apply settings 3" {
        n87 = local write "ACK 4"(FALSE ("Done")) -> ()
        n88 = Enqueue Element(queue=w218, element=T10 "C" ("Cmd"), error in (no error)=w217) -> (queue out=w215:refnum<queue>, error out=w216:errorcluster)  [unwired: 1 in, 1 out]
      }
      frame "Refresh system status" {
        n89 = Enqueue Element(queue=w223, element=T10 "G" ("Cmd"), error in (no error)=w224) -> (queue out=w226:refnum<queue>, error out=w227:errorcluster)  [unwired: 1 in, 1 out]
        n90 = local write "ACK 5"(FALSE ("ACK 8")) -> ()
        n91 = Enqueue Element(queue=w226, element=T10 "g" ("Cmd"), error in (no error)=w227) -> (queue out=w222:refnum<queue>, error out=w221:errorcluster)  [unwired: 1 in, 1 out]
      }
      frame Default {
        n92 = Enqueue Element(queue=w232, element=T10 "Exit" ("Cmd"), error in (no error)=w233) -> (queue out=w230:refnum<queue>, error out=w229:errorcluster)  [unwired: 1 in, 1 out]
      }
    }
    n93 = while {
      tunnel: w12 -> [w252]
      tunnel: w11 -> [w253]
      tunnel: [w240] -> w19
      shift-right: [w248] -> _
      shift-left: T9[] [] -> [w247]
      tunnel: [w244] -> w15
      tunnel: [w237] -> w13
      tunnel: [w236] -> w8
      tunnel: w6 -> [w235]
      tunnel: w5 -> [w234]
      stop <- w238 stop-if-true
      n94 = Dequeue Element(queue=w253, error in (no error)=w252) -> (queue out=w251:refnum<queue>, element=w249:T10, error out=w250:errorcluster)  [unwired: 1 in, 1 out]
      n95 = case shown="\"D\"" w249 {
        tunnel: w251 -> [w266 w279 w292 w337 w552 w564 w576 w588 w604 w625 w639 w649 w667 w686 w707 w729 w745 w746]
        tunnel: w250 -> [w265 w278 w291 w336 w551 w563 w575 w587 w603 w624 w638 w648 w666 w685 w706 w728 w744 w749]
        tunnel: [w263 w276 w289 w336 w551 w563 w575 w587 w603 w624 w638 w648 w666 w685 w706 w728 w744 w749] -> w242
        tunnel: [w262 w275 w288 w339 w550 w562 w574 w586 w602 w623 w637 w647 w665 w684 w687 w727 w743 errorcluster {"status"=FALSE, "code"=0, "source"=""} ("Error out")] -> w245
        tunnel: [w260 w273 w286 w338 w549 w561 w573 w585 w601 w622 w636 w646 w664 w683 w705 w726 w742 w747] -> w248
        tunnel: w247 -> [w260 w273 w286 w338 w549 w561 w573 w585 w601 w622 w636 w646 w664 w683 w704 w726 w742 w747]
        tunnel: [w264 w277 w290 w337 w552 w564 w576 w588 w604 w625 w639 w649 w667 w686 w707 w729 w745 w746] -> w243
        tunnel: [_ _ _ w335 _ _ _ _ _ _ _ _ _ _ _ _ _ _] -> w236
        tunnel: w235 -> [w259 w272 w285 w334 w547 w560 w565 w577 w589 w605 w630 w640 w650 w677 w688 w710 w730 _]
        tunnel: w234 -> [_ _ _ w333 w548 _ _ _ _ _ _ _ _ _ _ _ _ _]
        frame "P" {
          n96 = Enqueue Element At Opposite End(queue=w266, element=T10 "Busy" ("Cmd"), error in (no error)=w265) -> (queue out=w264:refnum<queue>, error out=w263:errorcluster)  [unwired: 1 in, 1 out]
          n97 = call "Open serial port.vi"("VISA resource name"=w259) -> ("Error out"=w257:errorcluster, "VISA resource name out"=w258:refnum<visa-resource-name>)  [unwired: 9 in]
          n98 = call "Power ON (P).vi"("Error In"=w257, "VISA resource name in"=w258) -> ("Error out"=w256:errorcluster, "ACK"=→"ACK 1":bool, "VISA resource name out"=w255:refnum<visa-resource-name>)  [unwired: 7 in]
          n99 = call "Close serial port.vi"("Error in"=w256, "VISA resource name"=w255) -> ("Error out"=w262:errorcluster)  [unwired: 9 in]
        }
        frame "p" {
          n100 = Enqueue Element At Opposite End(queue=w279, element=T10 "Busy" ("Cmd"), error in (no error)=w278) -> (queue out=w277:refnum<queue>, error out=w276:errorcluster)  [unwired: 1 in, 1 out]
          n101 = call "Open serial port.vi"("VISA resource name"=w272) -> ("Error out"=w270:errorcluster, "VISA resource name out"=w271:refnum<visa-resource-name>)  [unwired: 9 in]
          n102 = call "Power OFF (p).vi"("Error In"=w270, "VISA resource name in"=w271) -> ("Error out"=w269:errorcluster, "ACK"=w267:bool, "VISA resource name out"=w268:refnum<visa-resource-name>)  [unwired: 7 in]
          n103 = call "Close serial port.vi"("Error in"=w269, "VISA resource name"=w268) -> ("Error out"=w275:errorcluster)  [unwired: 9 in]
          n104 = local write "ACK 1"(w267) -> ()
        }
        frame "R" {
          n105 = Enqueue Element At Opposite End(queue=w292, element=T10 "Busy" ("Cmd"), error in (no error)=w291) -> (queue out=w290:refnum<queue>, error out=w289:errorcluster)  [unwired: 1 in, 1 out]
          n106 = call "Open serial port.vi"("VISA resource name"=w285) -> ("Error out"=w280:errorcluster, "VISA resource name out"=w281:refnum<visa-resource-name>)  [unwired: 9 in]
          n107 = call "Reset (R).vi"("Error In"=w280, "VISA resource name in"=w281) -> ("Error out"=w284:errorcluster, "ACK"=w282:bool, "VISA resource name out"=w283:refnum<visa-resource-name>)  [unwired: 7 in]
          n108 = call "Close serial port.vi"("Error in"=w284, "VISA resource name"=w283) -> ("Error out"=w288:errorcluster)  [unwired: 9 in]
          n109 = local write "ACK 1"(w282) -> ()
        }
        frame "S" {
          # "Env"
          # "P data Mode 1"
          # "P data Mode 0"
          # "Main streaming loop here, with display etc."
          n110 = local read "System status"() -> (w309:T6)
          n111 = local read "L_data (bytes)"() -> (w315:u16)
          n112 = property on="Stale samples flag" class="WFChart (strict)"("History Data"=u8[][] []) -> ()  [unwired: 2 in, 2 out]
          n113 = property on="Pressures time trace" class="WFChart (strict)"("History Data"=sgl[][] []) -> ()  [unwired: 2 in, 2 out]
          n114 = property on="Sensor temperatures time trace (Mode \"P & T\" only)" class="WFChart (strict)"("History Data"=sgl[][] []) -> ()  [unwired: 2 in, 2 out]
          n115 = case shown="False" "Wait for HW trigger" {
            tunnel: [w342 w346] -> w332
            tunnel: [w341 w347] -> w331
            tunnel: w334 -> [w340 w348]
            frame False {
              n116 = call "Open serial port.vi"("VISA resource name"=w340) -> ("Error out"=w343:errorcluster, "VISA resource name out"=w344:refnum<visa-resource-name>)  [unwired: 9 in]
              n117 = call "Start data stream (S).vi"("VISA resource name in"=w344, "Error In"=w343) -> ("VISA resource name out"=w341:refnum<visa-resource-name>, "Error out"=w342:errorcluster)  [unwired: 7 in]
            }
            frame True {
              n118 = call "Open serial port.vi"("timeout (ms)"=u32 4294967295, "VISA resource name"=w348) -> ("Error out"=w346:errorcluster, "VISA resource name out"=w347:refnum<visa-resource-name>)  [unwired: 8 in]
            }
          }
          n119 = local read "Env. period (ms)"() -> (w313:i32)
          n120 = Unbundle By Name(w309) -> ("Mode"=w299:u8)
          n121 = Decrement(x=w315) -> (x-1=w300:u16)
          n122 = Divide(x=2000.0 ("y"), y=w333) -> (x/y=w325:dbl)
          n123 = Divide(x=1000000.0 ("y"), y=w333) -> (x/y=w311:dbl)
          n124 = Divide(x=1000.0, y=w333) -> (x/y=w320:dbl)
          n125 = To Unsigned Long Integer(number=w300) -> (unsigned 32bit integer=w314:u32)
          n126 = Tick Count (ms)() -> (millisecond timer value=w301:u32)
          n127 = Get Date/Time In Seconds() -> (seconds since 1Jan1904=w330:timestamp)
          n128 = To Unsigned Long Integer(number=w320) -> (unsigned 32bit integer=w318:u32)
          n129 = To Unsigned Long Integer(number=w325) -> (unsigned 32bit integer=w324:u32)
          n130 = To Single Precision Float(number=w311) -> (single precision float=w310:sgl)
          n131 = while {
            shift-right: [w380] -> w328
            shift-left: w331 -> [w385]
            shift-right: [w379] -> w329
            shift-left: w332 -> [w386]
            tunnel: w330 -> [w378]
            tunnel: "Finite samples" -> [w375]
            tunnel: "N samples" -> [w377]
            shift-right: [w371] -> _
            shift-left: T9[] [] -> [w370]
            tunnel: w318 -> [w359]
            shift-right: [w366] -> _
            shift-left: T11[] [] -> [w368]
            shift-right: [w367] -> w335
            shift-left: T8[] [] -> [w369]
            tunnel: w314 -> [w365]
            tunnel: w313 -> [w364]
            tunnel: w310 -> [w363]
            tunnel: w299 -> [w352]
            shift-right: [w361] -> _
            shift-left: w301 -> [w360]
            shift-right: [w358] -> _
            shift-left: sgl[][] [] -> [w355]
            shift-right: [w357] -> _
            shift-left: u8[][] [] -> [w356]
            shift-right: [w354] -> _
            shift-left: sgl[][] [] -> [w353]
            shift-right: [w351] -> _
            shift-left: u32 1 ("x") -> [w350]
            tunnel: [FALSE] -> w293
            stop <- w372 stop-if-true
            # "stop if (((finite samples == true) && (i == Nsamples)) || (stop == true))"
            n132 = Equal?(x=w377, y=w350) -> (x = y?=w376:bool)
            n133 = VISA Read(VISA resource name=w385, byte count=u32 1, error in (no error)=w386) -> (VISA resource name out=w382:refnum<visa-resource-name>, read buffer=w383:string, error out=w381:errorcluster)  [unwired: 1 out]
            n134 = And(x=w375, y=w376) -> (x .and. y?=w373:bool)
            n135 = case shown="\"#\"" w383 {
              tunnel: w382 -> [w412 w527 w539]
              tunnel: w381 -> [w411 w526 w538]
              tunnel: [w409 w524 w539] -> w380
              tunnel: [w408 w525 w538] -> w379
              tunnel: w378 -> [w405 w521 _]
              tunnel: [w413 w520 w537] -> w371
              tunnel: w370 -> [w413 w519 w537]
              tunnel: w369 -> [w404 w516 w535]
              tunnel: w368 -> [w399 w515 w536]
              tunnel: [w403 w516 w535] -> w367
              tunnel: [w398 w515 w536] -> w366
              tunnel: w365 -> [w410 _ _]
              tunnel: w364 -> [_ w514 _]
              tunnel: w363 -> [w402 _ _]
              tunnel: [w401 FALSE ("Clock drift") FALSE ("Clock drift")] -> w362
              tunnel: w352 -> [w400 _ _]
              tunnel: [w397 w512 w533] -> w361
              tunnel: w360 -> [w396 w512 w533]
              tunnel: w359 -> [w395 _ _]
              tunnel: [w394 w510 w531] -> w358
              tunnel: w355 -> [w393 w510 w531]
              tunnel: [w392 w511 w532] -> w357
              tunnel: w356 -> [w391 w511 w532]
              tunnel: [w390 w509 w530] -> w354
              tunnel: w353 -> [w389 w509 w530]
              tunnel: [w388 w508 w529] -> w351
              tunnel: w350 -> [w387 w508 w529]
              frame "#" {
                # "Mode case"
                n136 = VISA Read(VISA resource name=w412, byte count=w410, error in (no error)=w411) -> (VISA resource name out=w409:refnum<visa-resource-name>, read buffer=w407:string, error out=w408:errorcluster)  [unwired: 1 out]
                n137 = local read "Active pressure sensor constants"() -> (w406:T7[])
                n138 = case shown="0, Default" w400 {
                  tunnel: w407 -> [w438 w481]
                  tunnel: w406 -> [w437 w480]
                  tunnel: w405 -> [w434 w477]
                  tunnel: w404 -> [w433 w482]
                  tunnel: [w432 w482] -> w403
                  tunnel: w402 -> [w431 w476]
                  tunnel: [w430 w475] -> w401
                  tunnel: w399 -> [w439 w474]
                  tunnel: [w439 w473] -> w398
                  tunnel: [w429 w468] -> w397
                  tunnel: w396 -> [w426 w464]
                  tunnel: w395 -> [w428 w465]
                  tunnel: [w424 w471] -> w394
                  tunnel: w393 -> [w423 w469]
                  tunnel: [w422 w472] -> w392
                  tunnel: w391 -> [w421 w470]
                  tunnel: [w420 w463] -> w390
                  tunnel: w389 -> [w420 w462]
                  frame 0, Default {
                    n139 = call "Process Data Buffer, Mode 0.vi"("DATA_Buffer excluding '#' [1...N]"=w438, "P constants"=w437) -> ("Pressures"=w415:sgl[], "Statuses"=w419:u8[], "dt_warn"=w435:u8)
                    n140 = Tick Count (ms)() -> (millisecond timer value=w418:u32)
                    n141 = Subtract(x=w418, y=w426) -> (x-y=w427:u32)
                    n142 = Greater Or Equal?(x=w427, y=w428) -> (x >= y?=w425:bool)
                    n143 = Array Size(array=w415) -> (size(s)=→"No Of Channels":i32)
                    n144 = Bundle By Name(cluster=T8 {"Time Stamp"=timestamp(3537581686.1176577 s since 1904-01-01), "dt (us)"=0.0, "dt_warn"=0, "Pressures"=[], "Statuses"=[]} ("P data (Mode 0)"), "Time Stamp"=w434, "dt (us)"=w431, "dt_warn"=w435, "Pressures"=w415, "Statuses"=w419) -> (w416:T8)
                    n145 = Type Cast(type=FALSE ("Clock drift"), x=w435) -> (*(type *) &x=w430:bool)
                    n146 = case shown="True" w425 {
                      tunnel: [w446 w455] -> w429
                      tunnel: w426 -> [w446 _]
                      tunnel: w418 -> [_ w455]
                      tunnel: w415 -> [w445 w453]
                      tunnel: [w444 sgl[][] []] -> w424
                      tunnel: w423 -> [w443 w454]
                      tunnel: w419 -> [w442 w450]
                      tunnel: [w441 u8[][] []] -> w422
                      tunnel: w421 -> [w440 w451]
                      frame False {
                        n147 = Build Array (concatenate)(w440, w442) -> (w441:u8[][])
                        n148 = Build Array (concatenate)(w443, w445) -> (w444:sgl[][])
                      }
                      frame True {
                        n149 = Build Array (concatenate)(w451, w450) -> (→"Stale samples flag":u8[][])
                        n150 = Build Array (concatenate)(w454, w453) -> (→"Pressures time trace":sgl[][])
                      }
                    }
                    n151 = Build Array (concatenate)(w433, w416) -> (w432:T8[])
                  }
                  frame 1 {
                    n152 = call "Process Data Buffer, Mode 1.vi"("DATA_Buffer excluding '#' [1...N]"=w481, "P constants"=w480) -> ("Pressures (Pa)"=w459:sgl[], "Sensor temps (degC)"=w461:sgl[], "Statuses"=w460:u8[], "dt_warn"=w478:u8)
                    n153 = Tick Count (ms)() -> (millisecond timer value=w458:u32)
                    n154 = Subtract(x=w458, y=w464) -> (x-y=w467:u32)
                    n155 = Greater Or Equal?(x=w467, y=w465) -> (x >= y?=w466:bool)
                    n156 = Bundle By Name(cluster=T11 {"Time Stamp"=timestamp(3537581686.1176577 s since 1904-01-01), "dt (us)"=0.0, "dt_warn"=0, "Pressures"=[], "Die temps."=[], "Statuses"=[]} ("P data (Mode 1)"), "Time Stamp"=w477, "dt (us)"=w476, "dt_warn"=w478, "Pressures"=w459, "Statuses"=w460, "Die temps."=w461) -> (w456:T11)
                    n157 = Type Cast(type=FALSE ("Clock drift"), x=w478) -> (*(type *) &x=w475:bool)
                    n158 = case shown="True" w466 {
                      tunnel: [w492 w505] -> w468
                      tunnel: w464 -> [w492 _]
                      tunnel: w458 -> [_ w505]
                      tunnel: w459 -> [w491 w503]
                      tunnel: [w490 sgl[][] []] -> w471
                      tunnel: w469 -> [w489 w504]
                      tunnel: w460 -> [w488 w500]
                      tunnel: [w487 u8[][] []] -> w472
                      tunnel: w470 -> [w486 w501]
                      tunnel: [w485 sgl[][] []] -> w463
                      tunnel: w461 -> [w484 w496]
                      tunnel: w462 -> [w483 w497]
                      frame False {
                        n159 = Build Array (concatenate)(w486, w488) -> (w487:u8[][])
                        n160 = Build Array (concatenate)(w489, w491) -> (w490:sgl[][])
                        n161 = Build Array (concatenate)(w483, w484) -> (w485:sgl[][])
                      }
                      frame True {
                        n162 = Build Array (concatenate)(w501, w500) -> (w494:u8[][])
                        n163 = Build Array (concatenate)(w504, w503) -> (w493:sgl[][])
                        n164 = Build Array (concatenate)(w497, w496) -> (→"Sensor temperatures time trace (Mode \"P & T\" only)":sgl[][])
                        n165 = local write "Stale samples flag"(w494) -> ()
                        n166 = local write "Pressures time trace"(w493) -> ()
                      }
                    }
                    n167 = Build Array (concatenate)(w474, w456) -> (w473:T11[])
                  }
                }
                n168 = Increment(x=w387) -> (x+1=w388:u32)
                "Samples acquired" <- w387
              }
              frame "$" {
                n169 = local read "AccelGyro constants"() -> (w522:T3)
                n170 = VISA Read(VISA resource name=w527, byte count=u32 29, error in (no error)=w526) -> (VISA resource name out=w524:refnum<visa-resource-name>, read buffer=w523:string, error out=w525:errorcluster)  [unwired: 1 out]
                n171 = call "Process State Buffer.vi"("AccelGyro constants"=w522, "STATE_Buffer excluding '$' [1...30]"=w523) -> ("Inertial state values"=w517:T4, "Environmental state values"=w518:T5)
                "Environmental state values" <- w518
                "Inertial state values" <- w517
                n172 = Bundle By Name(cluster=T9 {"Time Stamp"=timestamp(0 s since 1904-01-01), "dt (ms)"=0, "Environmental state values"={"Thermistor (degC)"=0.0, "Sensor temp. (degC)"=0.0, "P_atmos (Pa)"=0.0, "Rel. Humidity (%)"=0.0, "Density (kg/m^3)"=0.0, "Dew point (degC)"=0.0, "Pressure alt. (m)"=0.0, "Density alt. (m)"=0.0}, "Inertial state values"={"w_x (dps)"=0.0, "w_y (dps)"=0.0, "w_z (dps)"=0.0, "a_x (g)"=0.0, "a_y (g)"=0.0, "a_z (g)"=0.0, "Stale sample"=0, "Sensor temp. (degC)"=0.0}} ("All state values"), "Time Stamp"=w521, "dt (ms)"=w514, "Environmental state values"=w518, "Inertial state values"=w517) -> (w506:T9)
                n173 = Build Array (concatenate)(w519, w506) -> (w520:T9[])
              }
              frame Default {
              }
            }
            "Clock drift" <- w362
            n174 = Or(x="Stop streaming", y=w373) -> (x .or. y?=w372:bool)
          }
          n175 = Reciprocal(x=w333) -> (1/x=w308:dbl)
          n176 = property on="Pressures time trace" class="WFChart (strict)"("XScale.Multiplier"=w308) -> ()  [unwired: 2 in, 2 out]
          n177 = property on="Sensor temperatures time trace (Mode \"P & T\" only)" class="WFChart (strict)"("XScale.Multiplier"=w308) -> ()  [unwired: 2 in, 2 out]
          n178 = local write "Streaming"(w293) -> ()
          n179 = call "Stop data stream (s).vi"("VISA resource name in"=w328, "Error In"=w329) -> ("VISA resource name out"=w326:refnum<visa-resource-name>, "Error out"=w327:errorcluster)  [unwired: 7 in]
          n180 = call "Clear buffer.vi"("Error in"=w327, "dt for timeout (ms)"=w324, "VISA resource name in"=w326) -> ("Error out"=w296:errorcluster, "VISA resource name out"=w297:refnum<visa-resource-name>)  [unwired: 3 in]
          n181 = call "Close serial port.vi"("Error in"=w296, "VISA resource name"=w297) -> ("Error out"=w339:errorcluster)  [unwired: 9 in]
        }
        frame "T" {
          n182 = Divide(x=1000000.0, y=w548) -> (x/y=w541:dbl)
          n183 = call "Open serial port.vi"("VISA resource name"=w547) -> ("Error out"=w545:errorcluster, "VISA resource name out"=w546:refnum<visa-resource-name>)  [unwired: 9 in]
          n184 = call "Set stream dt (T).vi"("Error In"=w545, "dt (us)"=w541, "VISA resource name in"=w546) -> ("Error out"=w544:errorcluster, "ACK"=→"ACK 2":bool, "VISA resource name out"=w543:refnum<visa-resource-name>)  [unwired: 6 in]
          n185 = call "Close serial port.vi"("Error in"=w544, "VISA resource name"=w543) -> ("Error out"=w550:errorcluster)  [unwired: 9 in]
        }
        frame "t" {
          n186 = local read "Env. period (ms)"() -> (w554:i32)
          n187 = To Unsigned Long Integer(number=w554) -> (unsigned 32bit integer=w553:u32)
          n188 = call "Open serial port.vi"("VISA resource name"=w560) -> ("Error out"=w558:errorcluster, "VISA resource name out"=w559:refnum<visa-resource-name>)  [unwired: 9 in]
          n189 = call "Set state dt (t).vi"("Error In"=w558, "dt (ms)"=w553, "VISA resource name in"=w559) -> ("Error out"=w557:errorcluster, "ACK"=w555:bool, "VISA resource name out"=w556:refnum<visa-resource-name>)  [unwired: 6 in]
          n190 = call "Close serial port.vi"("Error in"=w557, "VISA resource name"=w556) -> ("Error out"=w562:errorcluster)  [unwired: 9 in]
          n191 = local write "ACK 2"(w555) -> ()
        }
        frame "M" {
          n192 = call "Open serial port.vi"("VISA resource name"=w565) -> ("Error out"=w571:errorcluster, "VISA resource name out"=w572:refnum<visa-resource-name>)  [unwired: 9 in]
          n193 = call "Set mode (M).vi"("Error In"=w571, "Mode"="Data mode", "VISA resource name in"=w572) -> ("Error out"=w570:errorcluster, "ACK"=w568:bool, "L_data"=→"L_data (bytes)":u16, "VISA resource name out"=w569:refnum<visa-resource-name>)  [unwired: 5 in]
          n194 = call "Close serial port.vi"("Error in"=w570, "VISA resource name"=w569) -> ("Error out"=w574:errorcluster)  [unwired: 9 in]
          n195 = local write "ACK 2"(w568) -> ()
        }
        frame "O" {
          n196 = call "Open serial port.vi"("VISA resource name"=w577) -> ("Error out"=w583:errorcluster, "VISA resource name out"=w584:refnum<visa-resource-name>)  [unwired: 9 in]
          n197 = call "Override maxSensorNum (O).vi"("Error In"=w583, "Max. number of sensors"="Max. num. sensors (override)", "VISA resource name in"=w584) -> ("Error out"=w582:errorcluster, "ACK"=→"ACK 3":bool, "L_data"=w578:u16, "VISA resource name out"=w581:refnum<visa-resource-name>)  [unwired: 5 in]
          n198 = local write "L_data (bytes)"(w578) -> ()
          n199 = call "Close serial port.vi"("Error in"=w582, "VISA resource name"=w581) -> ("Error out"=w586:errorcluster)  [unwired: 9 in]
        }
        frame "G" {
          n200 = call "Open serial port.vi"("VISA resource name"=w589) -> ("Error out"=w599:errorcluster, "VISA resource name out"=w600:refnum<visa-resource-name>)  [unwired: 9 in]
          n201 = call "Get status bits 1 (G).vi"("VISA resource name in"=w600, "Error In"=w599) -> ("nFaults"=w594:u8, "nSensors"=w593:u8, "nCards"=w592:u8, "PowerState"=w591:bool, "VISA resource name out"=w597:refnum<visa-resource-name>, "ACK"=→"ACK 5":bool, "Error out"=w598:errorcluster)  [unwired: 11 in]
          n202 = local read "System status"() -> (w590:T6)
          n203 = call "Close serial port.vi"("Error in"=w598, "VISA resource name"=w597) -> ("Error out"=w602:errorcluster)  [unwired: 9 in]
          n204 = Bundle By Name(cluster=w590, "Main power"=w591, "Occupied slots"=w592, "Active sensors"=w593, "Faulty sensors"=w594) -> (→"System status":T6)
        }
        frame "g" {
          w608 = T12."Disabled and Grayed Out" ("Disabled")
          w607 = T12."Enabled" ("Disabled")
          n205 = call "Open serial port.vi"("VISA resource name"=w605) -> ("Error out"=w620:errorcluster, "VISA resource name out"=w621:refnum<visa-resource-name>)  [unwired: 9 in]
          n206 = call "Get status bits 2 (g).vi"("VISA resource name in"=w621, "Error In"=w620) -> ("Mode"=w617:u8, "Therm_ok"=w609:bool, "BMI160_ok"=w613:bool, "BME280_ok"=w611:bool, "VISA resource name out"=w618:refnum<visa-resource-name>, "ACK"=w615:bool, "Error out"=w619:errorcluster)  [unwired: 11 in]
          n207 = Select(t=w607, s=w609, f=w608) -> (s? t:f=w612:T12)
          n208 = Select(t=w607, s=w611, f=w608) -> (s? t:f=w610:T12)
          n209 = stacked-sequence {
            tunnel: w612 -> [_ w627]
            tunnel: w610 -> [w626 _]
            tunnel: w609 -> [_ w628]
            frame #0 {
              n210 = property on="Environmental state values" class="Clust (strict)"("DisabledEnum"=w626) -> ()  [unwired: 2 in, 2 out]
              n211 = property on="Density (kg/m^3)" class="DigNum (strict)"("DisabledEnum"=w626) -> ()  [unwired: 2 in, 2 out]
              n212 = property on="Dew point (degC)" class="DigNum (strict)"("DisabledEnum"=w626) -> ()  [unwired: 2 in, 2 out]
              n213 = property on="Density alt. (m)" class="DigNum (strict)"("DisabledEnum"=w626) -> ()  [unwired: 2 in, 2 out]
            }
            frame #1 {
              n214 = case shown="False" w628 {
                tunnel: w627 -> [w629 _]
                frame False {
                  n215 = property on="Density (kg/m^3)" class="DigNum (strict)"("DisabledEnum"=w629) -> ()  [unwired: 2 in, 2 out]
                  n216 = property on="Dew point (degC)" class="DigNum (strict)"("DisabledEnum"=w629) -> ()  [unwired: 2 in, 2 out]
                  n217 = property on="Density alt. (m)" class="DigNum (strict)"("DisabledEnum"=w629) -> ()  [unwired: 2 in, 2 out]
                }
                frame True {
                }
              }
              n218 = property on="Thermistor (degC)" class="DigNum (strict)"("DisabledEnum"=w627) -> ()  [unwired: 2 in, 2 out]
            }
          }
          n219 = local read "System status"() -> (w614:T6)
          n220 = call "Close serial port.vi"("Error in"=w619, "VISA resource name"=w618) -> ("Error out"=w623:errorcluster)  [unwired: 9 in]
          n221 = local write "ACK 5"(w615) -> ()
          n222 = Select(t=w607, s=w613, f=w608) -> (s? t:f=w606:T12)
          n223 = Bundle By Name(cluster=w614, "Env. sensor"=w611, "Inertial sensor"=w613, "Thermistor"=w609, "Mode"=w617) -> (w616:T6)
          n224 = property on="Inertial state values" class="Clust (strict)"("DisabledEnum"=w606) -> ()  [unwired: 2 in, 2 out]
          n225 = property on="AccelGyro constants" class="Clust (strict)"("DisabledEnum"=w606) -> ()  [unwired: 2 in, 2 out]
          n226 = property on="Accel. range (g)" class="Ring (strict)"("DisabledEnum"=w606) -> ()  [unwired: 2 in, 2 out]
          n227 = property on="Accel. rate (Hz)" class="Ring (strict)"("DisabledEnum"=w606) -> ()  [unwired: 2 in, 2 out]
          n228 = property on="Gyro. range (dps)" class="Ring (strict)"("DisabledEnum"=w606) -> ()  [unwired: 2 in, 2 out]
          n229 = property on="Gyro. rate (Hz)" class="Ring (strict)"("DisabledEnum"=w606) -> ()  [unwired: 2 in, 2 out]
          n230 = property on="ACK 8" class="Bool (strict)"("DisabledEnum"=w606) -> ()  [unwired: 2 in, 2 out]
          n231 = local write "System status"(w616) -> ()
        }
        frame "F" {
          n232 = call "Open serial port.vi"("VISA resource name"=w630) -> ("Error out"=w634:errorcluster, "VISA resource name out"=w635:refnum<visa-resource-name>)  [unwired: 9 in]
          n233 = call "Collate faulty sensor indices.vi"("Error In"=w634, "VISA resource name in"=w635) -> ("Error out"=w633:errorcluster, "Faulty sensor indices"=→"Faulty sensors":i32[], "VISA resource name out"=w632:refnum<visa-resource-name>)  [unwired: 7 in]
          n234 = call "Close serial port.vi"("Error in"=w633, "VISA resource name"=w632) -> ("Error out"=w637:errorcluster)  [unwired: 9 in]
        }
        frame "A" {
          n235 = call "Open serial port.vi"("VISA resource name"=w640) -> ("Error out"=w644:errorcluster, "VISA resource name out"=w645:refnum<visa-resource-name>)  [unwired: 9 in]
          n236 = call "Collate active sensor indices.vi"("Error In"=w644, "VISA resource name in"=w645) -> ("Error out"=w643:errorcluster, "Active sensor indices"=→"Active sensors":i32[], "VISA resource name out"=w642:refnum<visa-resource-name>)  [unwired: 7 in]
          n237 = call "Close serial port.vi"("Error in"=w643, "VISA resource name"=w642) -> ("Error out"=w647:errorcluster)  [unwired: 9 in]
        }
        frame "C" {
          n238 = call "Open serial port.vi"("VISA resource name"=w650) -> ("Error out"=w662:errorcluster, "VISA resource name out"=w663:refnum<visa-resource-name>)  [unwired: 9 in]
          n239 = call "Configure BMI160 (C).vi"("VISA resource name in"=w663, "Accel. range (g)"="Accel. range (g)", "Accel. rate (Hz)"="Accel. rate (Hz)", "Gyro. range (dps)"="Gyro. range (dps)", "Gyro. rate (Hz)"="Gyro. rate (Hz)", "Error In"=w662) -> ("VISA resource name out"=w660:refnum<visa-resource-name>, "ACK ok"=→"ACK 4":bool, "Error out"=w661:errorcluster)  [unwired: 11 in]
          n240 = case shown="0, Default" "Accel. range (g)" {
            tunnel: [sgl 2.0 ("accRange") sgl 4.0 ("accRange") sgl 8.0 ("accRange") sgl 16.0 ("accRange")] -> w654
            frame 0, Default {
            }
            frame 1 {
            }
            frame 2 {
            }
            frame 3 {
            }
          }
          n241 = case shown="0, Default" "Gyro. range (dps)" {
            tunnel: [sgl 125.0 ("accRange") sgl 250.0 ("accRange") sgl 500.0 ("accRange") sgl 1000.0 ("accRange") sgl 2000.0 ("accRange")] -> w652
            frame 0, Default {
            }
            frame 1 {
            }
            frame 2 {
            }
            frame 3 {
            }
            frame 4 {
            }
          }
          n242 = call "Close serial port.vi"("Error in"=w661, "VISA resource name"=w660) -> ("Error out"=w665:errorcluster)  [unwired: 9 in]
          n243 = local read "AccelGyro constants"() -> (w651:T3)
          n244 = Bundle By Name(cluster=w651, "accRange"=w654, "gyrRange"=w652) -> (w656:T3)
          n245 = local write "AccelGyro constants"(w656) -> ()
        }
        frame "Z" {
          n246 = call "Open serial port.vi"("VISA resource name"=w677) -> ("Error out"=w681:errorcluster, "VISA resource name out"=w682:refnum<visa-resource-name>)  [unwired: 9 in]
          n247 = call "Get Serial Number (Z).vi"("VISA resource name in"=w682, "Error In"=w681) -> ("VISA resource name out"=w679:refnum<visa-resource-name>, "Serial Number"=→"Serial no.":u16, "Error out"=w680:errorcluster)  [unwired: 5 in, 1 out]
          n248 = call "Close serial port.vi"("Error in"=w680, "VISA resource name"=w679) -> ("Error out"=w684:errorcluster)  [unwired: 9 in]
        }
        frame "D" {
          # "write after interval has passed, else append"
          n249 = local read "AccelGyro constants"() -> (w696:T3)
          n250 = call "Open serial port.vi"("VISA resource name"=w688) -> ("Error out"=w702:errorcluster, "VISA resource name out"=w703:refnum<visa-resource-name>)  [unwired: 9 in]
          n251 = call "Get Env data (oneshot) (D).vi"("VISA resource name in"=w703, "Error In"=w702) -> ("VISA resource name out"=w700:refnum<visa-resource-name>, "STATE_Buffer"=w699:string, "ACK"=→"ACK 6":bool, "Error out"=w701:errorcluster)  [unwired: 5 in]
          n252 = local read "Env. period (ms)"() -> (w691:i32)
          n253 = Get Date/Time In Seconds() -> (seconds since 1Jan1904=w689:timestamp)
          n254 = call "Close serial port.vi"("Error in"=w701, "VISA resource name"=w700) -> ("Error out"=w687:errorcluster)  [unwired: 9 in]
          n255 = String Subset(string=w699, offset (0)=1) -> (substring=w698:string)  [unwired: 1 in]
          n256 = call "Process State Buffer.vi"("AccelGyro constants"=w696, "STATE_Buffer excluding '$' [1...30]"=w698) -> ("Inertial state values"=w693:T4, "Environmental state values"=w694:T5)
          n257 = Bundle By Name(cluster=T9 {"Time Stamp"=timestamp(0 s since 1904-01-01), "dt (ms)"=0, "Environmental state values"={"Thermistor (degC)"=0.0, "Sensor temp. (degC)"=0.0, "P_atmos (Pa)"=0.0, "Rel. Humidity (%)"=0.0, "Density (kg/m^3)"=0.0, "Dew point (degC)"=0.0, "Pressure alt. (m)"=0.0, "Density alt. (m)"=0.0}, "Inertial state values"={"w_x (dps)"=0.0, "w_y (dps)"=0.0, "w_z (dps)"=0.0, "a_x (g)"=0.0, "a_y (g)"=0.0, "a_z (g)"=0.0, "Stale sample"=0, "Sensor temp. (degC)"=0.0}} ("All state values"), "Time Stamp"=w689, "dt (ms)"=w691, "Environmental state values"=w694, "Inertial state values"=w693) -> (w690:T9)
          n258 = local write "Environmental state values"(w694) -> ()
          n259 = local write "Inertial state values"(w693) -> ()
          n260 = Build Array (concatenate)(w704, w690) -> (w705:T9[])
          n261 = case shown="No Error" w687 {
            frame No Error {
              n262 = global read "Pressure_Multiplexer_Server_Global.vi" "Acquisition Rendezvous Server"() -> (w708:T13)
              n263 = call <vilib>:"Wait at Rendezvous.vi"("ms timeout (-1)"=60000, "rendezvous"=w708) -> ()  [unwired: 3 in, 3 out]
            }
            frame Error {
            }
          }
        }
        frame "accgyr_consts" {
          (unwired) TRUE
          n264 = call "Open serial port.vi"("VISA resource name"=w710) -> ("Error out"=w724:errorcluster, "VISA resource name out"=w725:refnum<visa-resource-name>)  [unwired: 9 in]
          n265 = call "Get AccelGyro constants (MCU EEPROM).vi"("VISA resource name in"=w725, "Error In"=w724) -> ("VISA resource name out"=w722:refnum<visa-resource-name>, "AccelGyro constants"=w719:T3, "ACK"=→"ACK 8":bool, "Error out"=w723:errorcluster)  [unwired: 5 in]
          n266 = Unbundle By Name(w719) -> ("gx offset"=w718:sgl, "gy offset"=w717:sgl, "gz offset"=w716:sgl, "ax offset"=w715:sgl, "ay offset"=w714:sgl, "az offset"=w713:sgl, "axyz scale"=w712:sgl)
          n267 = call "Close serial port.vi"("Error in"=w723, "VISA resource name"=w722) -> ("Error out"=w727:errorcluster)  [unwired: 9 in]
          n268 = Bundle By Name(cluster=T3 {"gyrRange"=125.0, "accRange"=2.0, "gx offset"=0.0, "gy offset"=0.0, "gz offset"=0.0, "ax offset"=0.0, "ay offset"=0.0, "az offset"=0.0, "axyz scale"=1.0} ("AccelGyro constants"), "gx offset"=w718, "gy offset"=w717, "gz offset"=w716, "ax offset"=w715, "ay offset"=w714, "az offset"=w713, "axyz scale"=w712) -> (→"AccelGyro constants":T3)
        }
        frame "EEPROM_Pconsts" {
          # "Must only run this case after running \"P\", \"G\", \"A\""
          n269 = local read "System status"() -> (w735:T6)
          n270 = Unbundle By Name(w735) -> ("Occupied slots"=w734:u8)
          n271 = To Long Integer(number=w734) -> (32bit integer=w733:i32)
          n272 = call "Open serial port.vi"("VISA resource name"=w730) -> ("Error out"=w740:errorcluster, "VISA resource name out"=w741:refnum<visa-resource-name>)  [unwired: 9 in]
          n273 = local read "Active sensors"() -> (w737:i32[])
          n274 = call "Concatenate all slot EEPROM arrays.vi"("Error In"=w740, "N slots occupied"=w733, "VISA resource name in"=w741) -> ("Error out"=w739:errorcluster, "ACK (all)"=→"ACK 7":bool, "All slot EEPROM values"=w732:T14[], "VISA resource name out"=w738:refnum<visa-resource-name>)  [unwired: 5 in]
          n275 = call "Populate pressure constants array.vi"("Occupied slot EEPROM values"=w732, "Active sensor indices"=w737) -> ("Active pressure sensor constants"=→"Active pressure sensor constants":T7[])
          n276 = call "Close serial port.vi"("Error in"=w739, "VISA resource name"=w738) -> ("Error out"=w743:errorcluster)  [unwired: 9 in]
        }
        frame "Exit", Default {
          (unwired) FALSE
        }
      }
      n277 = Get Queue Status(queue=w243, return elements? (F)=FALSE, error in (no error)=w242) -> (queue out=w237:refnum<queue>, error out=w240:errorcluster, # elements in queue=w239:i32)  [unwired: 5 out]
      n278 = call <vilib>:"Clear Errors.vi"("error in (no error)"=w245, "specific error code to clear (0: all)"=1073676294) -> ("error out"=w244:errorcluster)  [unwired: 4 in, 1 out]
      "Error out" <- w244
      n279 = Equal To 0?(x=w239) -> (x = 0?=w238:bool)
    }
    "P data (mode 0)" <- w8
    n280 = Release Queue(queue=w13, error in (no error)=w19) -> (error out=w14:errorcluster)  [unwired: 1 in, 2 out]
    n281 = Merge Errors(w14, w15) -> (w16:errorcluster)
    n282 = local write "Error out"(w16) -> ()
    "Command" <- w4
  }
